vi "220221-VNA RP FLAT.vi"() -> ()   [LabVIEW 2021]
uses:
  b7fd31b3-4c8f-4ae8-a038-7c142e2eb182.vi
  <vilib>/Analysis/baseanly.llb/Mean (DBL).vi
  <vilib>/Utility/file.llb/Write Delimited Spreadsheet (DBL).vi
  <vilib>/Comparison/Equal/Equal Functor/Equal Functor.lvclass
  <vilib>/Analysis/NI_AALBase.lvlib
panel:
  in  "BTN VIEW PERSISTANCE":bool
  in  "Autoscale":bool
  in  "RP VNA SETTING":T1={"F start"=200000, "F stop"=2000500, "Sweep size"=1000, "Decimation"=5000, "F_corr"=0, "Ph_OUT1"=0, "Ph_OUT2"=0, "OUT_Lvl1"=32700, "OUT_Lvl2"=32700, "GPIO"=0}
  in  "Amplitude(1V)":dbl=0.3 format="%#_13g"
  out "RP CONNECT":bool
  in  "VOA Calibration cluster":cluster{"PUMP":dbl[], "PROBE":dbl[]}
  out "TRACK DATA REL NO SMOOTHING":dbl[][](array[numeric])
  out "TRACK DATA ABS NO SMOOTHING":dbl[][](array[numeric])
  in  "BTN SAVE TRACK":bool
  in  "BTN STOP TRACK":bool
  out "TRACK REPOSITERY":path
  out "TRACK DATA REL":dbl[][](array[numeric])
  out "TRACK DATA ABS":dbl[][](array[numeric])
  out "Track File List":path[](array[path])
  out "Track Repositery List":path[](array[path])
  out "CHANNEL CHOSEN":i32
  in  "TRACK-STOP":bool
  out "STATUS":string="STOP"
  out "track data":dbl[](array[numeric])=[495490.5081042979, 495481.56129759253, 495478.2328599854, 495479.84884744807, 495476.377462383, 495478.7819904735]
  out "Information tips":string
  in  "PANEL VNA":bool
  in  "PANEL TRACKING":bool
  in  "BTN STOP":bool
  in  "PANEL GENERAL SETTINGS":bool
  in  "PANEL TRACK SETTINGS":bool
  out "MAIN TAB":T2(tab)
  out "ACQ Indicator":bool
  in  "PUMP":dbl(slide)=100.0 min=0.0 max=100.0 step=0.1 scale=0.0..100.0
  in  "PROBE":dbl(slide)=100.0 min=0.0 max=100.0 step=0.1 scale=0.0..100.0
  in  "BTN RESET VNA":bool
  in  "SPAN":dbl=1900.0 format="%#5.1f"
  in  "STOP":dbl=2000.0 format="%#5.1f"
  in  "CENTER":dbl=1050.0 format="%#5.1f"
  in  "BTN AF VNA":bool
  out "MAGNITUDE/PHASE":cluster{cluster{dbl, dbl}[]}[](graph)
  in  "CHANNEL CHOICE VNA":T3(radio)
  in  "BTN Center to max":bool
  in  "BTN ZOOM-":bool
  in  "BTN ZOOM+":bool
  in  "START":dbl=200.0 format="%#5.1f"
  out "SPACING":dbl=1900.0 min=0.0 max=100.0 step=0.5 format="%#5.1f"
  in  "Points N°":i32=1000 min=600 max=5000 step=1 format="%#4.4g"
  in  "BTN LOOP VNA":bool
  in  "BTN RUN VNA":bool
  in  "BTN SAVE VNA":bool
  in  "Hide/Show track data channel":bool[](array[boolean])
  in  "BTN AUTOSAVE RAW DATA":bool=TRUE
  in  "COMMENTS":string
  in  "ASSAY NAME":string
  in  "DELAY AFTER SWITCH (s)":i32
  in  "N°POINTS TO DISPLAY":i32=200
  in  "DISPLAY OPTION":u16(ring) items=["Absolute frequency", "Relative frequency (ppm)"]
  in  "DELAY BETWEEN TRIG (s)":i32
  in  "AVERAGE/POINT":dbl=1.0
  out "LIVE TRACK":dbl[][](graph)
  out "CHANNELS IND TRACK":T3(radio)
  in  "BTN RUN TRACK":bool
  in  "TEMPORAL SMOOTHING":i32=15
  in  "BTN NEW TRACK":bool
  in  "BTN PAUSE TRACK":bool
  in  "CHANNELS PARAMETERS":T4(array[cluster])=[{"START 2"=200.0, "STOP 2"=2000.5, "CENTER 2"=1050.0, "SPAN 2"=1800.0, "CHANNEL TRACK ?"=FALSE, "PUMP"=100.0, "PROBE"=100.0, "Points N° 2"=1000, "SPACING 2"=100.0, "Parafit span"=0.0, "Parafit span type"=enum."Points N°"}, {"START 2"=200.0, "STOP 2"=2000.0, "CENTER 2"=1100.0, "SPAN 2"=1800.0, "CHANNEL TRACK ?"=FALSE, "PUMP"=100.0, "PROBE"=100.0, "Points N° 2"=1000, "SPACING 2"=1800.0, "Parafit span"=0.0, "Parafit span type"=enum."Points N°"}, {"START 2"=200.0, "STOP 2"=2000.0, "CENTER 2"=1100.0, "SPAN 2"=1800.0, "CHANNEL TRACK ?"=FALSE, "PUMP"=100.0, "PROBE"=100.0, "Points N° 2"=1000, "SPACING 2"=1800.0, "Parafit span"=0.0, "Parafit span type"=enum."Points N°"}, {"START 2"=200.0, "STOP 2"=2000.0, "CENTER 2"=1100.0, "SPAN 2"=1800.0, "CHANNEL TRACK ?"=FALSE, "PUMP"=100.0, "PROBE"=100.0, "Points N° 2"=1000, "SPACING 2"=1800.0, "Parafit span"=0.0, "Parafit span type"=enum."Points N°"}, {"START 2"=200.0, "STOP 2"=2000.0, "CENTER 2"=1100.0, "SPAN 2"=1800.0, "CHANNEL TRACK ?"=FALSE, "PUMP"=100.0, "PROBE"=100.0, "Points N° 2"=1000, "SPACING 2"=1800.0, "Parafit span"=0.0, "Parafit span type"=enum."Points N°"}, {"START 2"=200.0, "STOP 2"=2000.0, "CENTER 2"=1100.0, "SPAN 2"=1800.0, "CHANNEL TRACK ?"=FALSE, "PUMP"=100.0, "PROBE"=100.0, "Points N° 2"=1000, "SPACING 2"=1800.0, "Parafit span"=0.0, "Parafit span type"=enum."Points N°"}, {"START 2"=200.0, "STOP 2"=2000.0, "CENTER 2"=1100.0, "SPAN 2"=1800.0, "CHANNEL TRACK ?"=FALSE, "PUMP"=100.0, "PROBE"=100.0, "Points N° 2"=1000, "SPACING 2"=1800.0, "Parafit span"=0.0, "Parafit span type"=enum."Points N°"}, {"START 2"=200.0, "STOP 2"=2000.0, "CENTER 2"=1100.0, "SPAN 2"=1800.0, "CHANNEL TRACK ?"=FALSE, "PUMP"=100.0, "PROBE"=100.0, "Points N° 2"=1000, "SPACING 2"=1800.0, "Parafit span"=0.0, "Parafit span type"=enum."Points N°"}, {"START 2"=200.0, "STOP 2"=2000.0, "CENTER 2"=1100.0, "SPAN 2"=1800.0, "CHANNEL TRACK ?"=FALSE, "PUMP"=100.0, "PROBE"=100.0, "Points N° 2"=1000, "SPACING 2"=1800.0, "Parafit span"=0.0, "Parafit span type"=enum."Points N°"}, {"START 2"=200.0, "STOP 2"=2000.0, "CENTER 2"=1100.0, "SPAN 2"=1800.0, "CHANNEL TRACK ?"=FALSE, "PUMP"=100.0, "PROBE"=100.0, "Points N° 2"=1000, "SPACING 2"=1800.0, "Parafit span"=0.0, "Parafit span type"=enum."Points N°"}, {"START 2"=200.0, "STOP 2"=2000.0, "CENTER 2"=1100.0, "SPAN 2"=1800.0, "CHANNEL TRACK ?"=FALSE, "PUMP"=100.0, "PROBE"=100.0, "Points N° 2"=1000, "SPACING 2"=1800.0, "Parafit span"=0.0, "Parafit span type"=enum."Points N°"}, {"START 2"=200.0, "STOP 2"=2000.0, "CENTER 2"=1100.0, "SPAN 2"=1800.0, "CHANNEL TRACK ?"=FALSE, "PUMP"=100.0, "PROBE"=100.0, "Points N° 2"=1000, "SPACING 2"=1800.0, "Parafit span"=0.0, "Parafit span type"=enum."Points N°"}, {"START 2"=200.0, "STOP 2"=2000.0, "CENTER 2"=1100.0, "SPAN 2"=1800.0, "CHANNEL TRACK ?"=FALSE, "PUMP"=100.0, "PROBE"=100.0, "Points N° 2"=1000, "SPACING 2"=1800.0, "Parafit span"=0.0, "Parafit span type"=enum."Points N°"}, {"START 2"=200.0, "STOP 2"=2000.0, "CENTER 2"=1100.0, "SPAN 2"=1800.0, "CHANNEL TRACK ?"=FALSE, "PUMP"=100.0, "PROBE"=100.0, "Points N° 2"=1000, "SPACING 2"=1800.0, "Parafit span"=0.0, "Parafit span type"=enum."Points N°"}, {"START 2"=200.0, "STOP 2"=2000.0, "CENTER 2"=1100.0, "SPAN 2"=1800.0, "CHANNEL TRACK ?"=FALSE, "PUMP"=100.0, "PROBE"=100.0, "Points N° 2"=1000, "SPACING 2"=1800.0, "Parafit span"=0.0, "Parafit span type"=enum."Points N°"}, {"START 2"=200.0, "STOP 2"=2000.0, "CENTER 2"=1100.0, "SPAN 2"=1800.0, "CHANNEL TRACK ?"=FALSE, "PUMP"=100.0, "PROBE"=100.0, "Points N° 2"=1000, "SPACING 2"=1800.0, "Parafit span"=0.0, "Parafit span type"=enum."Points N°"}] {"SPACING 2" min=0.0 max=100.0 step=0.5; "Points N° 2" min=0 max=100 step=1; "PROBE" min=0.0 max=100.0 step=0.5; "PUMP" min=0.0 max=100.0 step=0.5}
  out "CHANNEL IND SETTINGS":T5(radio)
  in  "TRACK DATA PARAMETERS":cluster{"MAIN FOLDER":path}={"MAIN FOLDER"=path "C:/SensWay Data"}
  in  "SPECTRUM POST PROCESSING PARAMETERS":cluster{"N° SMOOTHING POINTS":i32}={"N° SMOOTHING POINTS"=50}
  in  "AUTOFOCUS PARAMETERS":cluster{"ITERATIONS":i32}={"ITERATIONS"=5}
  in  "CHANNELS":T6
  in  "NETWORK PARAMETERS":T7={"RP-IP 1"="192.168.0.3", "RP-IP 2"="192.168.0.4", "RP-MAC 1"="", "RP-MAC 2"=""}
  in  "PERSISTANCE DATA CLUSTER":T8
  in  "VNA DATA CLUSTER":T8
  in  "TRACK DATA CLUSTER":cluster{"CHANNEL":dbl, "KPI 1 TRACK":ext[]}
  out "LOOP ACT":bool
  out "RAW Freq table":dbl[](array[numeric])=[200000.0, 201802.3023023023, 203604.6046046046, 205406.9069069069, 207209.20920920922, 209011.51151151152, 210813.81381381382, 212616.1161161161, 214418.4184184184, 216220.7207207207, 218023.02302302304, 219825.32532532534, 221627.62762762763, 223429.92992992993, 225232.23223223223, 227034.53453453453, 228836.83683683682, 230639.13913913915, 232441.44144144145, 234243.74374374375, 236046.04604604605, 237848.34834834834, 239650.65065065064, 241452.95295295294, 243255.25525525527, 245057.55755755756, 246859.85985985986, 248662.16216216216, 250464.46446446446, 252266.76676676676, 254069.06906906905, 255871.37137137138, 257673.67367367368, 259475.97597597598, 261278.27827827827, 263080.5805805806, 264882.8828828829, 266685.18518518517, 268487.4874874875, 270289.7897897898, 272092.0920920921, 273894.39439439436, 275696.6966966967, 277498.998998999, 279301.3013013013, 281103.6036036036, 282905.9059059059, 284708.2082082082, 286510.51051051053, 288312.8128128128, 290115.1151151151, 291917.4174174174, 293719.7197197197, 295522.02202202205, 297324.3243243243, 299126.6266266266, 300928.9289289289, 302731.23123123124, 304533.5335335335, 306335.83583583584, 308138.1381381381, 309940.44044044043, 311742.74274274276, 313545.04504504503, 315347.34734734736, 317149.6496496496, 318951.95195195195, 320754.2542542543, 322556.55655655655, 324358.8588588588, 326161.16116116114, 327963.4634634635, 329765.76576576574, 331568.06806806807, 333370.37037037034, 335172.67267267266, 336974.974974975, 338777.27727727726, 340579.5795795796, 342381.88188188185, 344184.1841841842, 345986.4864864865, 347788.7887887888, 349591.09109109105, 351393.3933933934, 353195.6956956957, 354997.997997998, 356800.3003003003, 358602.60260260256, 360404.9049049049, 362207.2072072072, 364009.50950950955, 365811.8118118118, 367614.1141141141, 369416.4164164164, 371218.71871871874, 373021.021021021, 374823.3233233233, 376625.6256256256, 378427.9279279279, 380230.23023023026, 382032.5325325325, 383834.8348348348, 385637.1371371371, 387439.43943943945, 389241.7417417418, 391044.04404404404, 392846.3463463463, 394648.64864864864, 396450.95095095097, 398253.25325325324, 400055.5555555555, 401857.85785785783, 403660.16016016016, 405462.4624624625, 407264.76476476475, 409067.067067067, 410869.36936936935, 412671.6716716717, 414473.973973974, 416276.2762762763, 418078.57857857854, 419880.88088088087, 421683.1831831832, 423485.48548548546, 425287.7877877878, 427090.09009009006, 428892.3923923924, 430694.6946946947, 432496.996996997, 434299.29929929925, 436101.6016016016, 437903.9039039039, 439706.20620620623, 441508.5085085085, 443310.81081081077, 445113.1131131131, 446915.4154154154, 448717.7177177177, 450520.02002002, 452322.3223223223, 454124.6246246246, 455926.92692692694, 457729.2292292292, 459531.5315315315, 461333.8338338338, 463136.13613613613, 464938.4384384384, 466740.74074074073, 468543.04304304306, 470345.3453453453, 472147.64764764765, 473949.9499499499, 475752.25225225225, 477554.5545545545, 479356.85685685684, 481159.1591591592, 482961.46146146144, 484763.76376376377, 486566.06606606604, 488368.36836836836, 490170.67067067063, 491972.97297297296, 493775.2752752753, 495577.57757757755, 497379.8798798799, 499182.18218218215, 500984.4844844845, 502786.78678678675, 504589.0890890891, 506391.3913913914, 508193.69369369367, 509995.995995996, 511798.29829829826, 513600.6006006006, 515402.90290290286, 517205.2052052052, 519007.5075075075, 520809.8098098098, 522612.1121121121, 524414.4144144144, 526216.7167167168, 528019.0190190191, 529821.3213213213, 531623.6236236236, 533425.9259259258, 535228.2282282282, 537030.5305305305, 538832.8328328328, 540635.1351351351, 542437.4374374375, 544239.7397397398, 546042.042042042, 547844.3443443443, 549646.6466466465, 551448.9489489489, 553251.2512512512, 555053.5535535535, 556855.8558558559, 558658.1581581582, 560460.4604604605, 562262.7627627627, 564065.065065065, 565867.3673673674, 567669.6696696696, 569471.9719719719, 571274.2742742742, 573076.5765765766, 574878.8788788789, 576681.1811811812, 578483.4834834835, 580285.7857857858, 582088.0880880881, 583890.3903903903, 585692.6926926926, 587494.994994995, 589297.2972972973, 591099.5995995996, 592901.9019019019, 594704.2042042043, 596506.5065065065, 598308.8088088088, 600111.111111111, 601913.4134134133, 603715.7157157157, 605518.018018018, 607320.3203203203, 609122.6226226226, 610924.924924925, 612727.2272272272, 614529.5295295295, 616331.8318318318, 618134.134134134, 619936.4364364364, 621738.7387387387, 623541.041041041, 625343.3433433434, 627145.6456456457, 628947.947947948, 630750.2502502502, 632552.5525525525, 634354.8548548548, 636157.1571571571, 637959.4594594594, 639761.7617617617, 641564.0640640641, 643366.3663663664, 645168.6686686687, 646970.9709709709, 648773.2732732733, 650575.5755755756, 652377.8778778778, 654180.1801801801, 655982.4824824824, 657784.7847847848, 659587.0870870871, 661389.3893893894, 663191.6916916918, 664993.993993994, 666796.2962962963, 668598.5985985985, 670400.9009009008, 672203.2032032032, 674005.5055055055, 675807.8078078078, 677610.1101101101, 679412.4124124125, 681214.7147147147, 683017.017017017, 684819.3193193192, 686621.6216216215, 688423.9239239239, 690226.2262262262, 692028.5285285285, 693830.8308308308, 695633.1331331332, 697435.4354354354, 699237.7377377377, 701040.04004004, 702842.3423423423, 704644.6446446446, 706446.9469469469, 708249.2492492492, 710051.5515515516, 711853.8538538539, 713656.1561561562, 715458.4584584584, 717260.7607607607, 719063.063063063, 720865.3653653653, 722667.6676676676, 724469.9699699699, 726272.2722722723, 728074.5745745746, 729876.8768768768, 731679.1791791791, 733481.4814814815, 735283.7837837838, 737086.0860860861, 738888.3883883883, 740690.6906906907, 742492.992992993, 744295.2952952953, 746097.5975975975, 747899.8998998998, 749702.2022022022, 751504.5045045045, 753306.8068068068, 755109.109109109, 756911.4114114114, 758713.7137137137, 760516.016016016, 762318.3183183183, 764120.6206206206, 765922.9229229229, 767725.2252252252, 769527.5275275275, 771329.8298298299, 773132.1321321321, 774934.4344344344, 776736.7367367367, 778539.039039039, 780341.3413413413, 782143.6436436436, 783945.9459459459, 785748.2482482482, 787550.5505505506, 789352.8528528528, 791155.1551551551, 792957.4574574574, 794759.7597597598, 796562.0620620621, 798364.3643643643, 800166.6666666666, 801968.968968969, 803771.2712712713, 805573.5735735735, 807375.8758758758, 809178.1781781781, 810980.4804804805, 812782.7827827828, 814585.085085085, 816387.3873873873, 818189.6896896897, 819991.991991992, 821794.2942942943, 823596.5965965965, 825398.8988988989, 827201.2012012012, 829003.5035035035, 830805.8058058057, 832608.108108108, 834410.4104104104, 836212.7127127127, 838015.015015015, 839817.3173173172, 841619.6196196196, 843421.9219219219, 845224.2242242242, 847026.5265265265, 848828.8288288288, 850631.1311311311, 852433.4334334334, 854235.7357357357, 856038.0380380381, 857840.3403403403, 859642.6426426426, 861444.9449449449, 863247.2472472473, 865049.5495495495, 866851.8518518518, 868654.1541541541, 870456.4564564564, 872258.7587587588, 874061.061061061, 875863.3633633633, 877665.6656656656, 879467.967967968, 881270.2702702703, 883072.5725725725, 884874.8748748748, 886677.1771771772, 888479.4794794795, 890281.7817817817, 892084.084084084, 893886.3863863864, 895688.6886886887, 897490.990990991, 899293.2932932932, 901095.5955955955, 902897.8978978979, 904700.2002002002, 906502.5025025025, 908304.8048048047, 910107.1071071071, 911909.4094094094, 913711.7117117117, 915514.0140140139, 917316.3163163163, 919118.6186186186, 920920.9209209209, 922723.2232232232, 924525.5255255254, 926327.8278278278, 928130.1301301301, 929932.4324324324, 931734.7347347348, 933537.037037037, 935339.3393393393, 937141.6416416416, 938943.943943944, 940746.2462462463, 942548.5485485485, 944350.8508508508, 946153.1531531531, 947955.4554554555, 949757.7577577577, 951560.06006006, 953362.3623623623, 955164.6646646647, 956966.966966967, 958769.2692692692, 960571.5715715715, 962373.8738738738, 964176.1761761762, 965978.4784784785, 967780.7807807807, 969583.083083083, 971385.3853853854, 973187.6876876877, 974989.9899899899, 976792.2922922922, 978594.5945945946, 980396.8968968969, 982199.1991991992, 984001.5015015014, 985803.8038038037, 987606.1061061061, 989408.4084084084, 991210.7107107107, 993013.0130130129, 994815.3153153153, 996617.6176176176, 998419.9199199199, 1000222.2222222221, 1002024.5245245245, 1003826.8268268268, 1005629.1291291291, 1007431.4314314314, 1009233.7337337337, 1011036.036036036, 1012838.3383383383, 1014640.6406406406, 1016442.942942943, 1018245.2452452452, 1020047.5475475475, 1021849.8498498498, 1023652.1521521521, 1025454.4544544544, 1027256.7567567567, 1029059.059059059, 1030861.3613613613, 1032663.6636636637, 1034465.9659659659, 1036268.2682682682, 1038070.5705705705, 1039872.8728728729, 1041675.1751751752, 1043477.4774774774, 1045279.7797797797, 1047082.082082082, 1048884.3843843844, 1050686.6866866867, 1052488.988988989, 1054291.2912912914, 1056093.5935935937, 1057895.895895896, 1059698.198198198, 1061500.5005005004, 1063302.8028028028, 1065105.105105105, 1066907.4074074074, 1068709.7097097095, 1070512.0120120118, 1072314.3143143142, 1074116.6166166165, 1075918.9189189188, 1077721.2212212211, 1079523.5235235235, 1081325.8258258258, 1083128.1281281281, 1084930.4304304305, 1086732.7327327328, 1088535.035035035, 1090337.3373373374, 1092139.6396396398, 1093941.9419419419, 1095744.2442442442, 1097546.5465465465, 1099348.8488488488, 1101151.1511511512, 1102953.4534534533, 1104755.7557557556, 1106558.058058058, 1108360.3603603602, 1110162.6626626626, 1111964.964964965, 1113767.2672672672, 1115569.5695695695, 1117371.8718718719, 1119174.1741741742, 1120976.4764764765, 1122778.7787787789, 1124581.0810810812, 1126383.3833833835, 1128185.6856856856, 1129987.987987988, 1131790.2902902903, 1133592.5925925926, 1135394.894894895, 1137197.197197197, 1138999.4994994993, 1140801.8018018017, 1142604.104104104, 1144406.4064064063, 1146208.7087087086, 1148011.011011011, 1149813.3133133133, 1151615.6156156156, 1153417.917917918, 1155220.2202202203, 1157022.5225225226, 1158824.824824825, 1160627.1271271273, 1162429.4294294294, 1164231.7317317317, 1166034.034034034, 1167836.3363363363, 1169638.6386386384, 1171440.9409409408, 1173243.243243243, 1175045.5455455454, 1176847.8478478477, 1178650.15015015, 1180452.4524524524, 1182254.7547547547, 1184057.057057057, 1185859.3593593594, 1187661.6616616617, 1189463.963963964, 1191266.2662662663, 1193068.5685685687, 1194870.8708708708, 1196673.173173173, 1198475.4754754754, 1200277.7777777778, 1202080.08008008, 1203882.3823823822, 1205684.6846846845, 1207486.9869869868, 1209289.2892892892, 1211091.5915915915, 1212893.8938938938, 1214696.1961961961, 1216498.4984984985, 1218300.8008008008, 1220103.103103103, 1221905.4054054054, 1223707.7077077078, 1225510.01001001, 1227312.3123123124, 1229114.6146146145, 1230916.9169169168, 1232719.2192192192, 1234521.5215215215, 1236323.8238238238, 1238126.126126126, 1239928.4284284282, 1241730.7307307306, 1243533.033033033, 1245335.3353353352, 1247137.6376376376, 1248939.9399399399, 1250742.2422422422, 1252544.5445445445, 1254346.8468468469, 1256149.1491491492, 1257951.4514514515, 1259753.7537537536, 1261556.056056056, 1263358.3583583583, 1265160.6606606606, 1266962.962962963, 1268765.2652652652, 1270567.5675675676, 1272369.86986987, 1274172.1721721722, 1275974.4744744743, 1277776.7767767766, 1279579.079079079, 1281381.3813813813, 1283183.6836836836, 1284985.985985986, 1286788.2882882883, 1288590.5905905906, 1290392.892892893, 1292195.195195195, 1293997.4974974974, 1295799.7997997997, 1297602.102102102, 1299404.4044044043, 1301206.7067067067, 1303009.009009009, 1304811.3113113113, 1306613.6136136136, 1308415.915915916, 1310218.218218218, 1312020.5205205204, 1313822.8228228227, 1315625.125125125, 1317427.4274274274, 1319229.7297297297, 1321032.032032032, 1322834.3343343344, 1324636.6366366367, 1326438.9389389388, 1328241.241241241, 1330043.5435435434, 1331845.8458458458, 1333648.148148148, 1335450.4504504504, 1337252.7527527527, 1339055.055055055, 1340857.3573573574, 1342659.6596596597, 1344461.9619619618, 1346264.2642642641, 1348066.5665665665, 1349868.8688688688, 1351671.1711711711, 1353473.4734734735, 1355275.7757757758, 1357078.078078078, 1358880.3803803804, 1360682.6826826825, 1362484.9849849849, 1364287.2872872872, 1366089.5895895895, 1367891.8918918918, 1369694.1941941942, 1371496.4964964965, 1373298.7987987988, 1375101.1011011011, 1376903.4034034032, 1378705.7057057056, 1380508.008008008, 1382310.3103103102, 1384112.6126126125, 1385914.9149149149, 1387717.2172172172, 1389519.5195195195, 1391321.8218218219, 1393124.1241241242, 1394926.4264264263, 1396728.7287287286, 1398531.031031031, 1400333.3333333333, 1402135.6356356356, 1403937.937937938, 1405740.2402402402, 1407542.5425425426, 1409344.844844845, 1411147.147147147, 1412949.4494494493, 1414751.7517517516, 1416554.054054054, 1418356.3563563563, 1420158.6586586586, 1421960.960960961, 1423763.2632632633, 1425565.5655655656, 1427367.867867868, 1429170.17017017, 1430972.4724724723, 1432774.7747747747, 1434577.077077077, 1436379.3793793793, 1438181.6816816817, 1439983.983983984, 1441786.2862862863, 1443588.5885885886, 1445390.8908908907, 1447193.193193193, 1448995.4954954954, 1450797.7977977977, 1452600.1001001, 1454402.4024024024, 1456204.7047047047, 1458007.007007007, 1459809.3093093093, 1461611.6116116114, 1463413.9139139138, 1465216.216216216, 1467018.5185185184, 1468820.8208208208, 1470623.123123123, 1472425.4254254254, 1474227.7277277277, 1476030.03003003, 1477832.3323323324, 1479634.6346346345, 1481436.9369369368, 1483239.2392392391, 1485041.5415415415, 1486843.8438438438, 1488646.146146146, 1490448.4484484484, 1492250.7507507508, 1494053.053053053, 1495855.3553553552, 1497657.6576576575, 1499459.9599599598, 1501262.2622622622, 1503064.5645645645, 1504866.8668668668, 1506669.1691691692, 1508471.4714714715, 1510273.7737737738, 1512076.0760760761, 1513878.3783783782, 1515680.6806806806, 1517482.9829829829, 1519285.2852852852, 1521087.5875875875, 1522889.8898898899, 1524692.1921921922, 1526494.4944944945, 1528296.7967967968, 1530099.099099099, 1531901.4014014013, 1533703.7037037036, 1535506.006006006, 1537308.3083083082, 1539110.6106106106, 1540912.912912913, 1542715.2152152152, 1544517.5175175176, 1546319.8198198196, 1548122.122122122, 1549924.4244244243, 1551726.7267267266, 1553529.029029029, 1555331.3313313313, 1557133.6336336336, 1558935.935935936, 1560738.2382382383, 1562540.5405405406, 1564342.8428428427, 1566145.145145145, 1567947.4474474473, 1569749.7497497497, 1571552.052052052, 1573354.3543543543, 1575156.6566566566, 1576958.958958959, 1578761.2612612613, 1580563.5635635634, 1582365.8658658657, 1584168.168168168, 1585970.4704704704, 1587772.7727727727, 1589575.075075075, 1591377.3773773774, 1593179.6796796797, 1594981.981981982, 1596784.2842842843, 1598586.5865865864, 1600388.8888888888, 1602191.191191191, 1603993.4934934934, 1605795.7957957957, 1607598.098098098, 1609400.4004004004, 1611202.7027027027, 1613005.005005005, 1614807.3073073071, 1616609.6096096095, 1618411.9119119118, 1620214.2142142141, 1622016.5165165165, 1623818.8188188188, 1625621.121121121, 1627423.4234234234, 1629225.7257257258, 1631028.0280280279, 1632830.3303303302, 1634632.6326326325, 1636434.9349349348, 1638237.2372372372, 1640039.5395395395, 1641841.8418418418, 1643644.1441441441, 1645446.4464464465, 1647248.7487487488, 1649051.051051051, 1650853.3533533532, 1652655.6556556555, 1654457.9579579579, 1656260.2602602602, 1658062.5625625625, 1659864.8648648649, 1661667.1671671672, 1663469.4694694695, 1665271.7717717716, 1667074.074074074, 1668876.3763763763, 1670678.6786786786, 1672480.980980981, 1674283.2832832832, 1676085.5855855856, 1677887.887887888, 1679690.1901901902, 1681492.4924924925, 1683294.7947947946, 1685097.097097097, 1686899.3993993993, 1688701.7017017016, 1690504.004004004, 1692306.3063063063, 1694108.6086086086, 1695910.910910911, 1697713.2132132133, 1699515.5155155153, 1701317.8178178177, 1703120.12012012, 1704922.4224224223, 1706724.7247247247, 1708527.027027027, 1710329.3293293293, 1712131.6316316316, 1713933.933933934, 1715736.236236236, 1717538.5385385384, 1719340.8408408407, 1721143.143143143, 1722945.4454454454, 1724747.7477477477, 1726550.05005005, 1728352.3523523523, 1730154.6546546547, 1731956.956956957, 1733759.259259259, 1735561.5615615614, 1737363.8638638637, 1739166.166166166, 1740968.4684684684, 1742770.7707707707, 1744573.073073073, 1746375.3753753754, 1748177.6776776777, 1749979.9799799798, 1751782.2822822821, 1753584.5845845845, 1755386.8868868868, 1757189.189189189, 1758991.4914914914, 1760793.7937937938, 1762596.096096096, 1764398.3983983984, 1766200.7007007005, 1768003.0030030028, 1769805.3053053052, 1771607.6076076075, 1773409.9099099098, 1775212.2122122122, 1777014.5145145145, 1778816.8168168168, 1780619.1191191191, 1782421.4214214215, 1784223.7237237236, 1786026.0260260259, 1787828.3283283282, 1789630.6306306305, 1791432.9329329329, 1793235.2352352352, 1795037.5375375375, 1796839.8398398398, 1798642.1421421422, 1800444.4444444443, 1802246.7467467466, 1804049.049049049, 1805851.3513513512, 1807653.6536536536, 1809455.955955956, 1811258.2582582582, 1813060.5605605606, 1814862.8628628629, 1816665.1651651652, 1818467.4674674673, 1820269.7697697696, 1822072.072072072, 1823874.3743743743, 1825676.6766766766, 1827478.978978979, 1829281.2812812813, 1831083.5835835836, 1832885.885885886, 1834688.188188188, 1836490.4904904903, 1838292.7927927927, 1840095.095095095, 1841897.3973973973, 1843699.6996996996, 1845502.002002002, 1847304.3043043043, 1849106.6066066066, 1850908.9089089087, 1852711.211211211, 1854513.5135135134, 1856315.8158158157, 1858118.118118118, 1859920.4204204204, 1861722.7227227227, 1863525.025025025, 1865327.3273273273, 1867129.6296296297, 1868931.9319319318, 1870734.234234234, 1872536.5365365364, 1874338.8388388387, 1876141.141141141, 1877943.4434434434, 1879745.7457457457, 1881548.048048048, 1883350.3503503504, 1885152.6526526525, 1886954.9549549548, 1888757.2572572571, 1890559.5595595594, 1892361.8618618618, 1894164.164164164, 1895966.4664664664, 1897768.7687687688, 1899571.071071071, 1901373.3733733734, 1903175.6756756755, 1904977.9779779778, 1906780.2802802802, 1908582.5825825825, 1910384.8848848848, 1912187.1871871871, 1913989.4894894895, 1915791.7917917918, 1917594.0940940941, 1919396.3963963962, 1921198.6986986985, 1923001.0010010009, 1924803.3033033032, 1926605.6056056055, 1928407.9079079079, 1930210.2102102102, 1932012.5125125125, 1933814.8148148148, 1935617.117117117, 1937419.4194194193, 1939221.7217217216, 1941024.024024024, 1942826.3263263262, 1944628.6286286286, 1946430.930930931, 1948233.2332332332, 1950035.5355355355, 1951837.8378378379, 1953640.14014014, 1955442.4424424423, 1957244.7447447446, 1959047.047047047, 1960849.3493493493, 1962651.6516516516, 1964453.953953954, 1966256.2562562563, 1968058.5585585586, 1969860.8608608607, 1971663.163163163, 1973465.4654654653, 1975267.7677677677, 1977070.07007007, 1978872.3723723723, 1980674.6746746746, 1982476.976976977, 1984279.2792792793, 1986081.5815815816, 1987883.8838838837, 1989686.186186186, 1991488.4884884884, 1993290.7907907907, 1995093.093093093, 1996895.3953953953, 1998697.6976976977, 2000500.0]
  in  "ENABLE INTERNAL MODULATION":bool=TRUE
  in  "VNA DATA CLUSTER TBL":T9(array[cluster])=[{"CHANNEL"=0.0, "FREQUENCY TABLE"=[0.0], "MAGNITUDE TABLE"=[0.0], "PHASE TABLE"=[0.0]}, {"CHANNEL"=1.0, "FREQUENCY TABLE"=[], "MAGNITUDE TABLE"=[], "PHASE TABLE"=[]}, {"CHANNEL"=2.0, "FREQUENCY TABLE"=[], "MAGNITUDE TABLE"=[], "PHASE TABLE"=[]}, {"CHANNEL"=3.0, "FREQUENCY TABLE"=[], "MAGNITUDE TABLE"=[], "PHASE TABLE"=[]}, {"CHANNEL"=4.0, "FREQUENCY TABLE"=[], "MAGNITUDE TABLE"=[], "PHASE TABLE"=[]}, {"CHANNEL"=5.0, "FREQUENCY TABLE"=[], "MAGNITUDE TABLE"=[], "PHASE TABLE"=[]}, {"CHANNEL"=6.0, "FREQUENCY TABLE"=[], "MAGNITUDE TABLE"=[], "PHASE TABLE"=[]}, {"CHANNEL"=7.0, "FREQUENCY TABLE"=[], "MAGNITUDE TABLE"=[], "PHASE TABLE"=[]}, {"CHANNEL"=8.0, "FREQUENCY TABLE"=[], "MAGNITUDE TABLE"=[], "PHASE TABLE"=[]}, {"CHANNEL"=9.0, "FREQUENCY TABLE"=[], "MAGNITUDE TABLE"=[], "PHASE TABLE"=[]}, {"CHANNEL"=10.0, "FREQUENCY TABLE"=[], "MAGNITUDE TABLE"=[], "PHASE TABLE"=[]}, {"CHANNEL"=11.0, "FREQUENCY TABLE"=[], "MAGNITUDE TABLE"=[], "PHASE TABLE"=[]}, {"CHANNEL"=12.0, "FREQUENCY TABLE"=[], "MAGNITUDE TABLE"=[], "PHASE TABLE"=[]}, {"CHANNEL"=13.0, "FREQUENCY TABLE"=[], "MAGNITUDE TABLE"=[], "PHASE TABLE"=[]}, {"CHANNEL"=14.0, "FREQUENCY TABLE"=[], "MAGNITUDE TABLE"=[], "PHASE TABLE"=[]}, {"CHANNEL"=15.0, "FREQUENCY TABLE"=[], "MAGNITUDE TABLE"=[], "PHASE TABLE"=[]}]
  in  "TRACK DATA CLUSTER TBL":cluster{"CHANNEL":dbl, "KPI 1 TRACK":ext[]}[](array[cluster])
  in  "VNA Settings cluster":T10={"START 2"=200.0, "STOP 2"=2000.5, "CENTER 2"=1050.0, "SPAN 2"=1901.0, "CHANNEL TRACK ?"=FALSE, "PUMP"=100.0, "PROBE"=100.0, "Points N° 2"=1000, "SPACING 2"=1901.0, "Parafit span"=0.0, "Parafit span type"=enum."Points N°"} {"SPACING 2" min=0.0 max=100.0 step=0.5; "Points N° 2" min=0 max=100 step=1; "PROBE" min=0.0 max=100.0 step=0.5; "PUMP" min=0.0 max=100.0 step=0.5}
  # "E"
  # "POINTS"
  # "SPACING"
  # "TRACK ?"
  # "START"
  # "STOP"
  # "CENTER"
  # "SPAN"
  # "PROBE"
  # "PUMP"
  # "PARABOLIC FIT SPAN"
  # "DATA ENTRY"
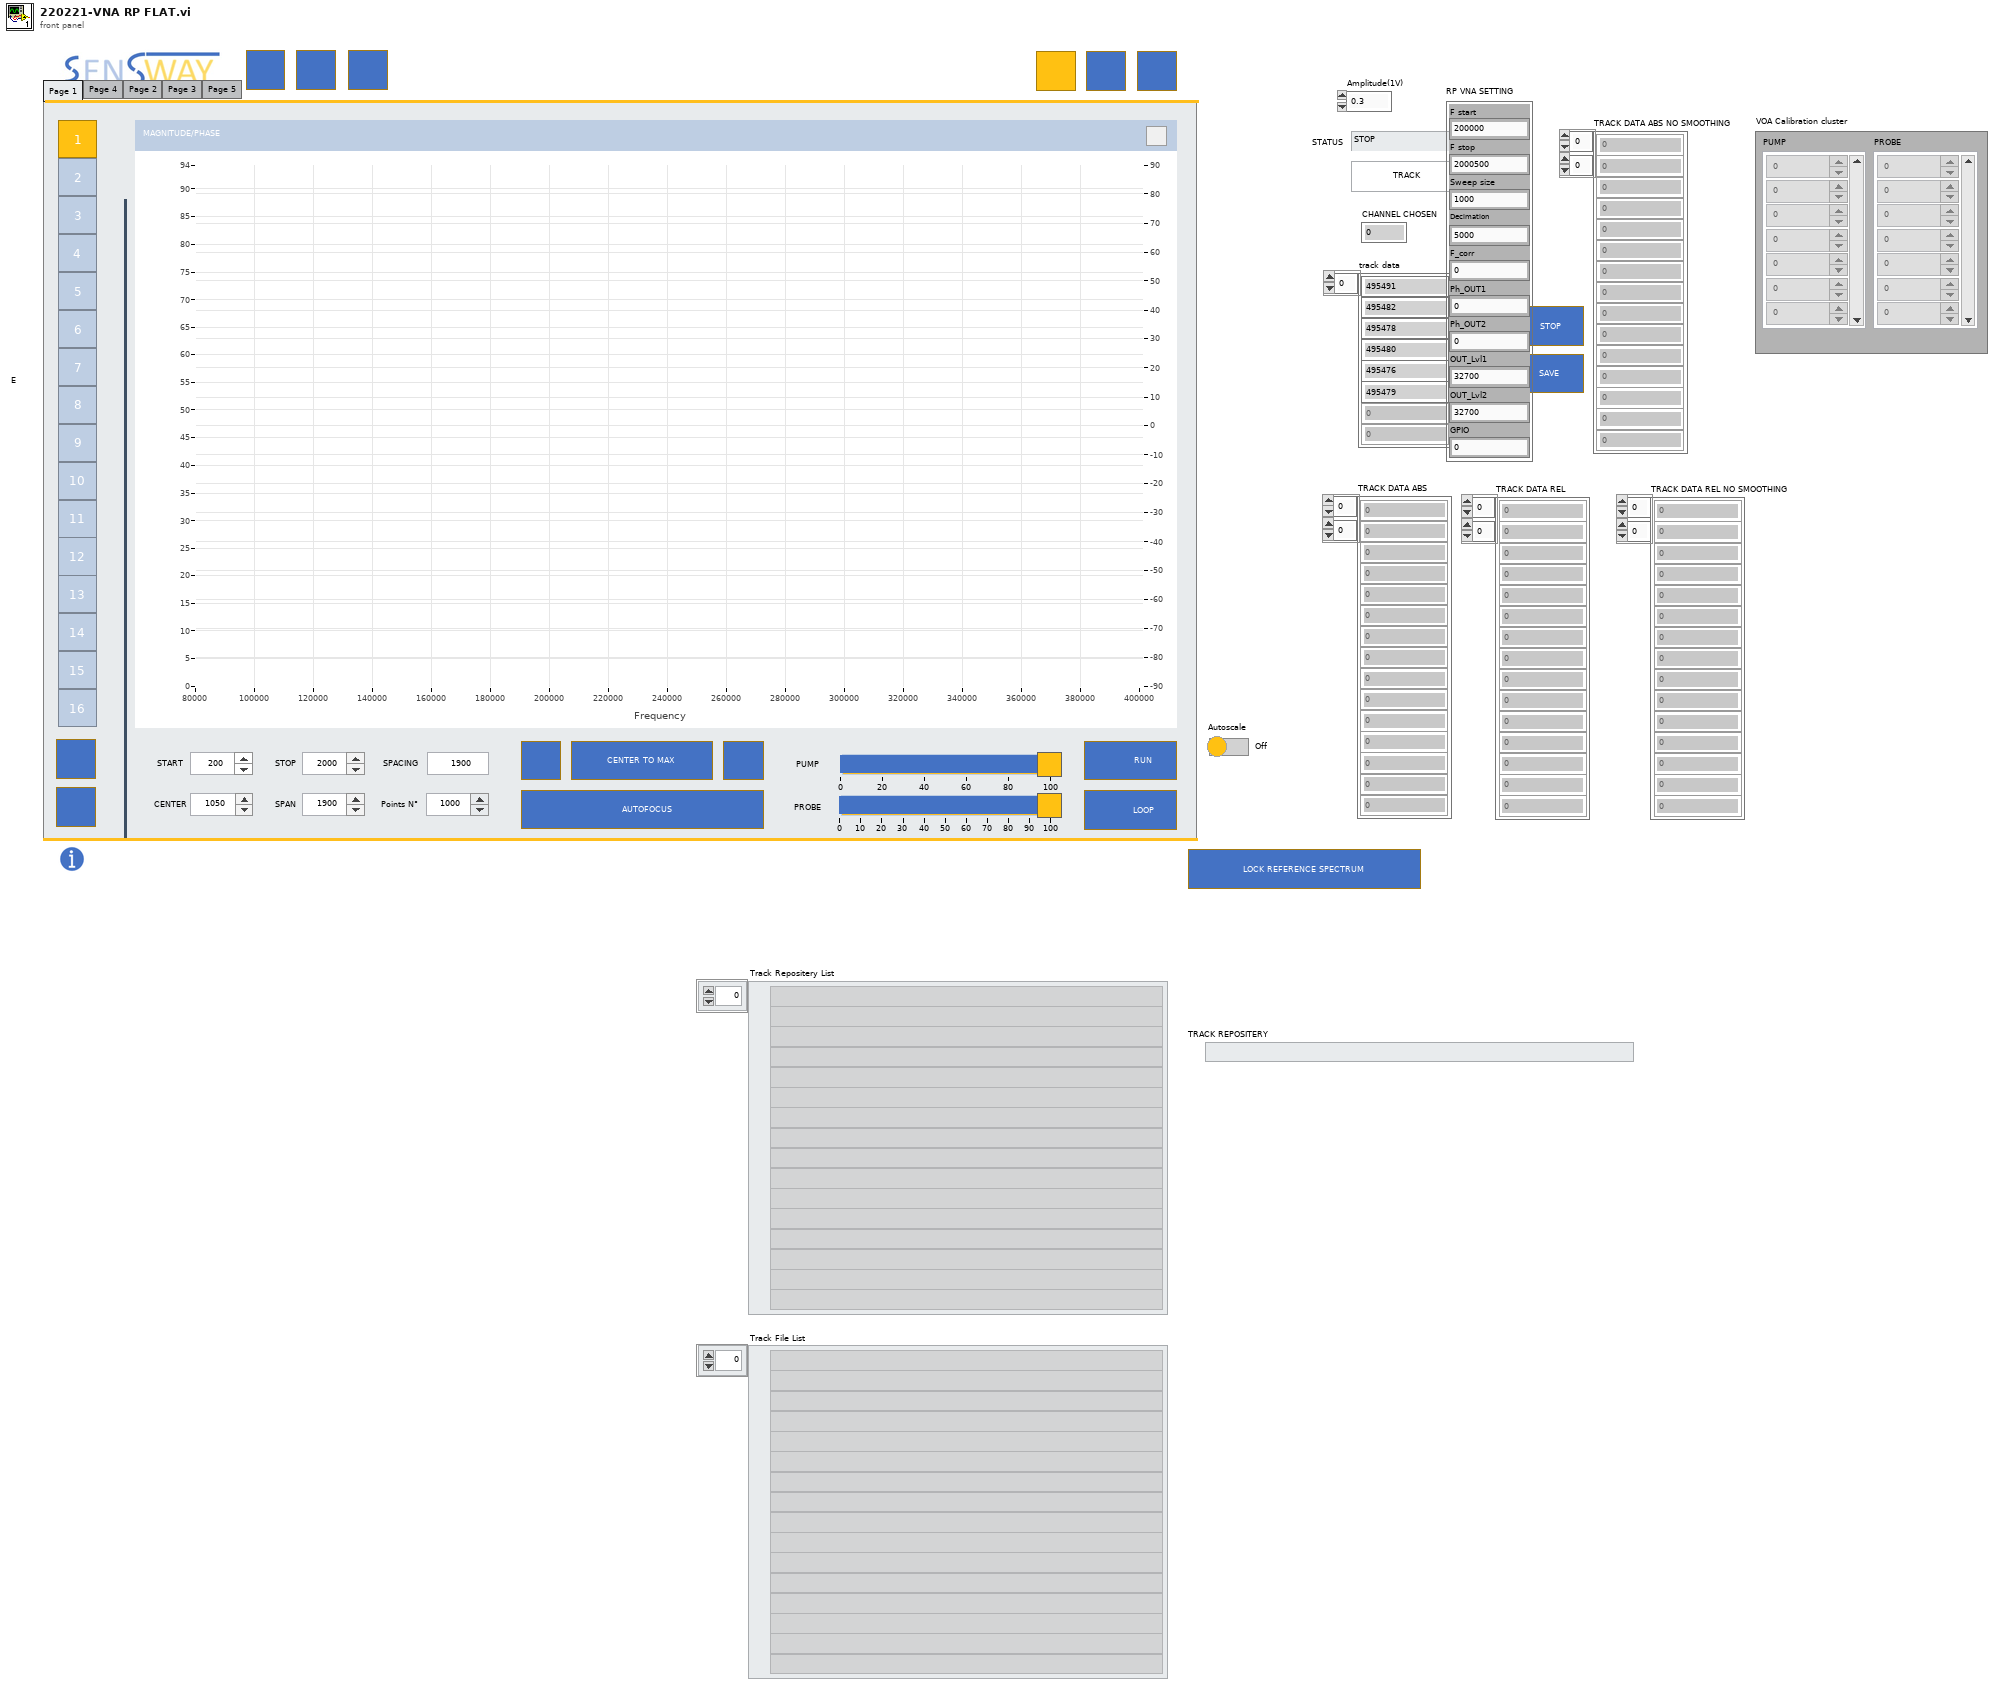
[diagram p1: front panel]
types:
  T1 = cluster{"F start":u32, "F stop":u32, "Sweep size":u32, "Decimation":u32, "F_corr":u32, "Ph_OUT1":u32, "Ph_OUT2":u32, "OUT_Lvl1":u32, "OUT_Lvl2":u32, "GPIO":u32}
  T2 = enum32{"Page 1", "Page 4", "Page 2", "Page 3", "Page 5"}
  T3 = enum32{"Button 1", "Button 2", "Button 3", "Sélection radio 4", "Sélection radio 5", "Sélection radio 6", "Sélection radio 7", "Sélection radio 8", "Sélection radio 9", "Sélection radio 10", "Sélection radio 11", "Sélection radio 12", "Sélection radio 13", "Sélection radio 14", "Sélection radio 15", "Sélection radio 16"}
  T4 = cluster{"START 2":dbl, "STOP 2":dbl, "CENTER 2":dbl, "SPAN 2":dbl, "CHANNEL TRACK ?":bool, "PUMP":dbl, "PROBE":dbl, "Points N° 2":i32, "SPACING 2":dbl, "Parafit span":dbl, "Parafit span type":enum16{"Points N°", "Frequency", "Span %"}}[]
  T5 = enum32{"No Selection", "Button 1", "Button 2", "Button 3", "Sélection radio 4", "Sélection radio 5", "Sélection radio 6", "Sélection radio 7", "Sélection radio 8", "Sélection radio 9", "Sélection radio 10", "Sélection radio 11", "Sélection radio 12", "Sélection radio 13", "Sélection radio 14", "Sélection radio 15", "Sélection radio 16"}
  T6 = cluster{"CHANNEL 1":bool, "CHANNEL 2":bool, "CHANNEL 3":bool, "CHANNEL 4":bool, "CHANNEL 5":bool, "CHANNEL 6":bool, "CHANNEL 7":bool, "CHANNEL 8":bool, "CHANNEL 9":bool, "CHANNEL 10":bool, "CHANNEL 11":bool, "CHANNEL 12":bool, "CHANNEL 13":bool, "CHANNEL 14":bool, "CHANNEL 15":bool, "CHANNEL 16":bool}
  T7 = cluster{"RP-IP 1":string, "RP-IP 2":string, "RP-MAC 1":string, "RP-MAC 2":string}
  T8 = cluster{"CHANNEL":dbl, "FREQUENCY TABLE":ext[], "MAGNITUDE TABLE":ext[], "PHASE TABLE":ext[]}
  T9 = cluster{"CHANNEL":dbl, "FREQUENCY TABLE":ext[], "MAGNITUDE TABLE":ext[], "PHASE TABLE":ext[]}[]
  T10 = cluster{"START 2":dbl, "STOP 2":dbl, "CENTER 2":dbl, "SPAN 2":dbl, "CHANNEL TRACK ?":bool, "PUMP":dbl, "PROBE":dbl, "Points N° 2":i32, "SPACING 2":dbl, "Parafit span":dbl, "Parafit span type":enum16{"Points N°", "Frequency", "Span %"}}
  T11 = enum16{"Freq start", "Freq stop", "Sweep size", "Decimation rate", "Freq corr", "Phase output 1", "Phase output 2", "Output level 1", "Output level 2", "GPIO", "SWEEP START"}
  T12 = cluster{"Numeric Control":ext, "Numeric Control":ext}[]
  T13 = cluster{cluster{"Numeric Control":ext, "Numeric Control":ext}[]}
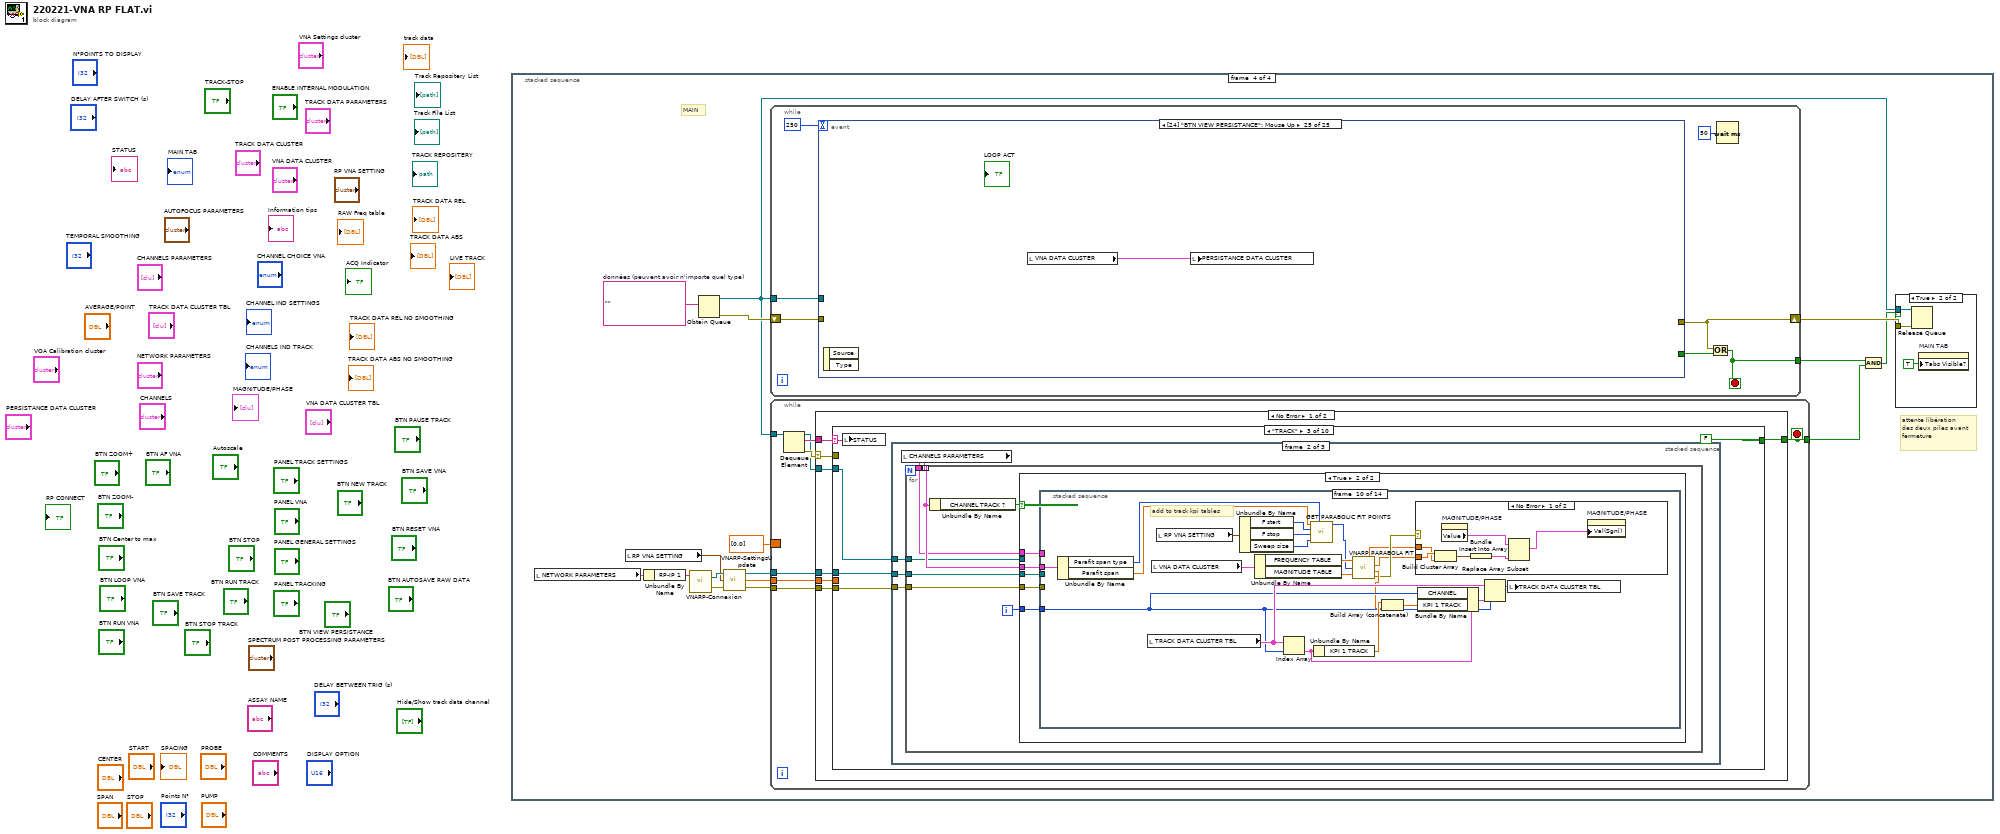
[diagram p0: block diagram]
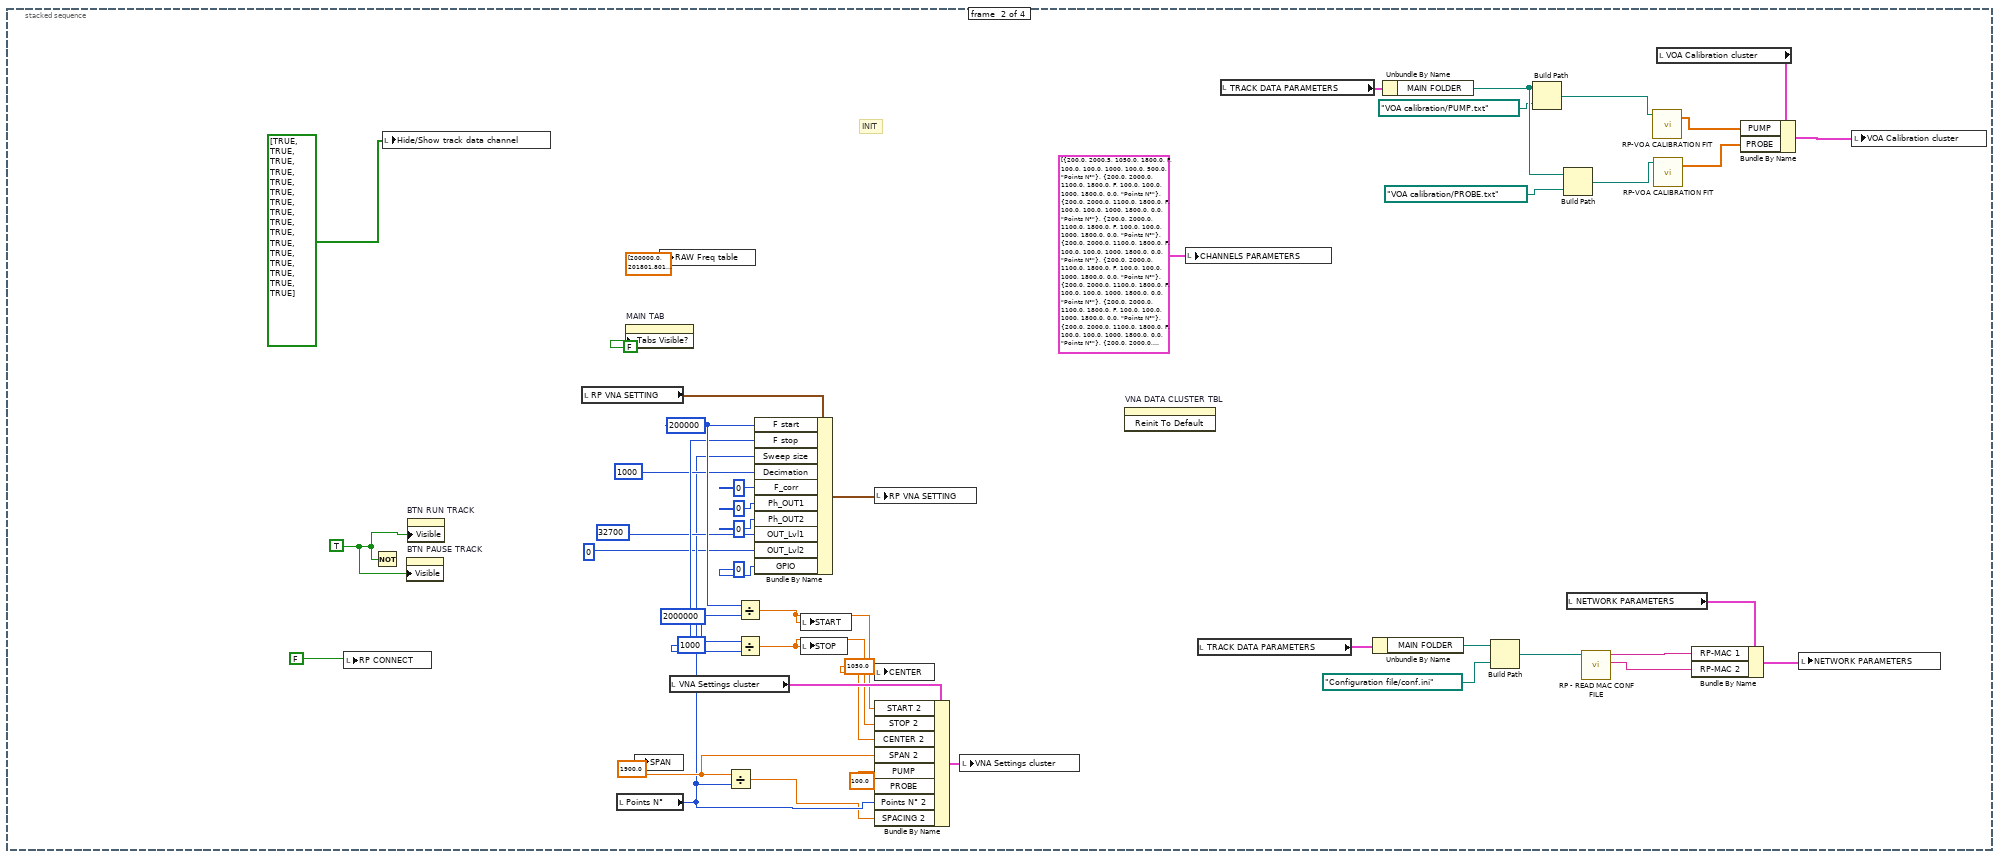
[diagram p3: hidden frame]
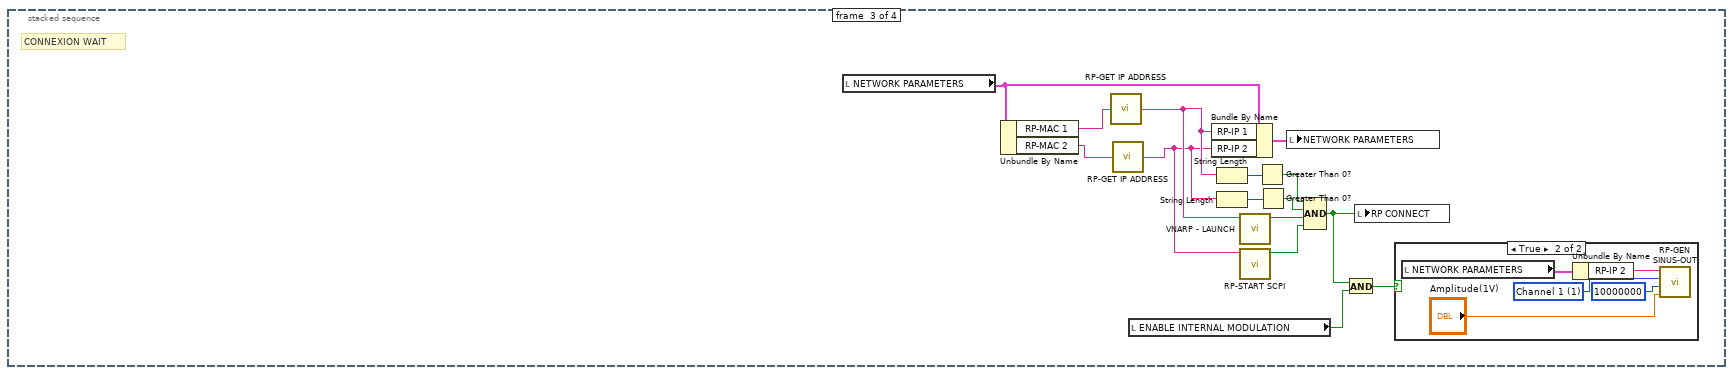
[diagram p4: hidden frame]
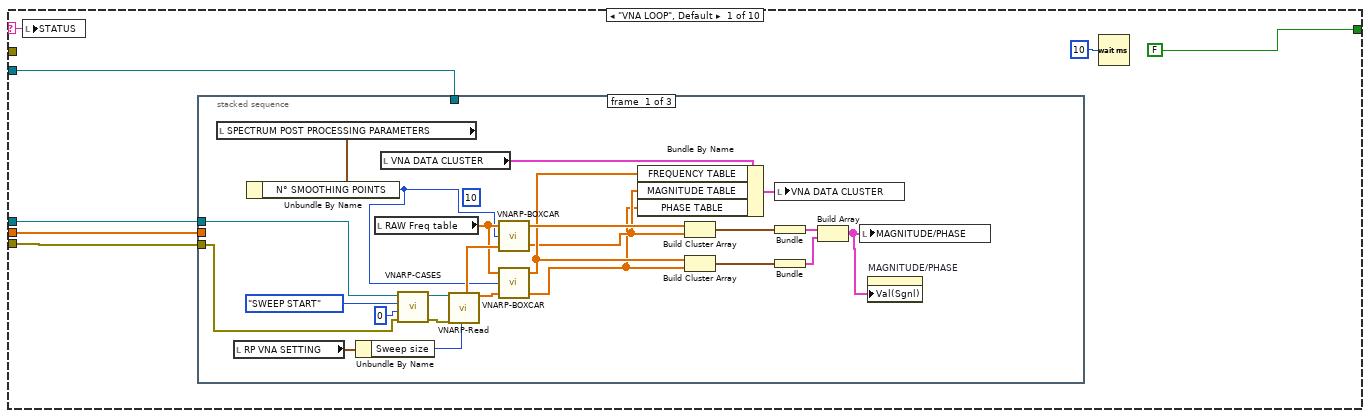
[diagram p7: hidden frame]
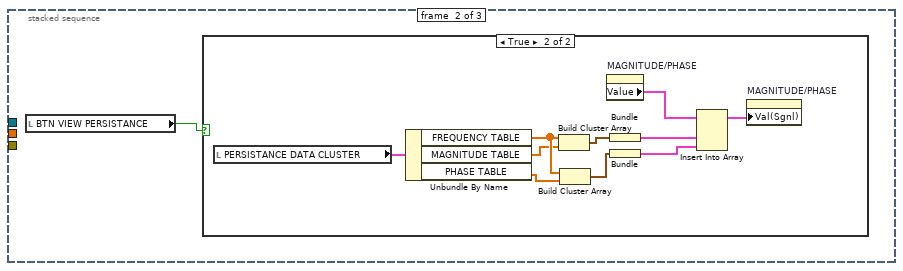
[diagram p8: hidden frame]
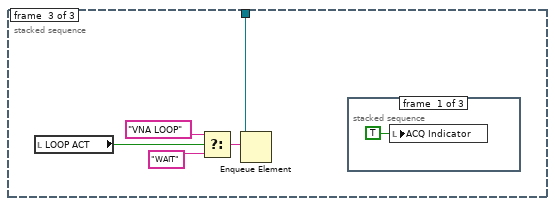
[diagram p10: hidden frame]
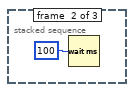
[diagram p11: hidden frame]
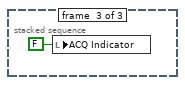
[diagram p12: hidden frame]
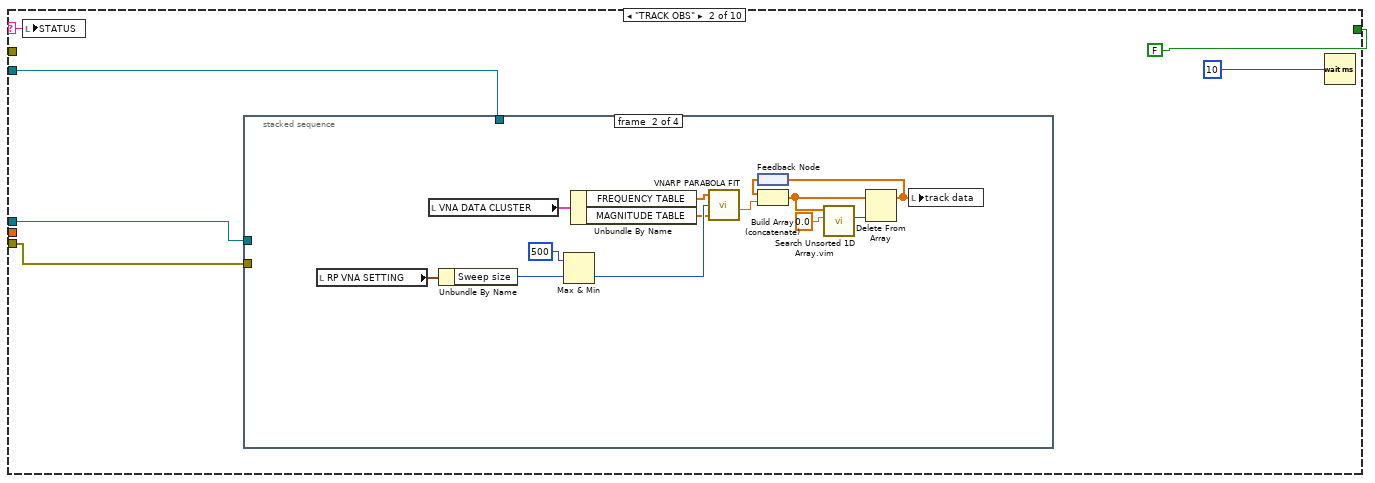
[diagram p13: hidden frame]
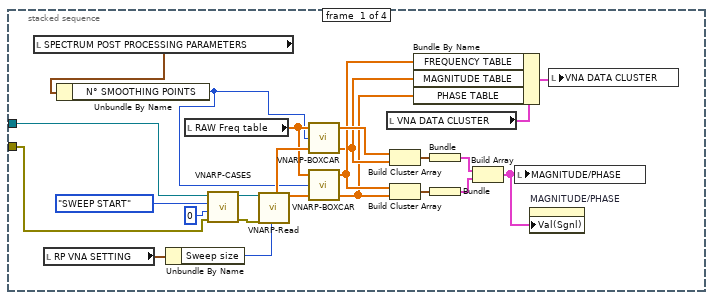
[diagram p14: hidden frame]
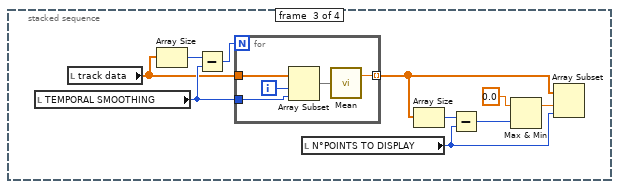
[diagram p15: hidden frame]
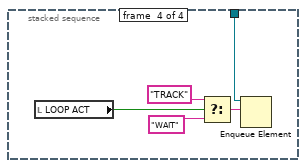
[diagram p16: hidden frame]
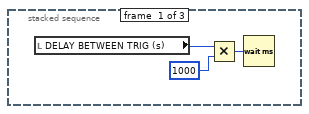
[diagram p17: hidden frame]
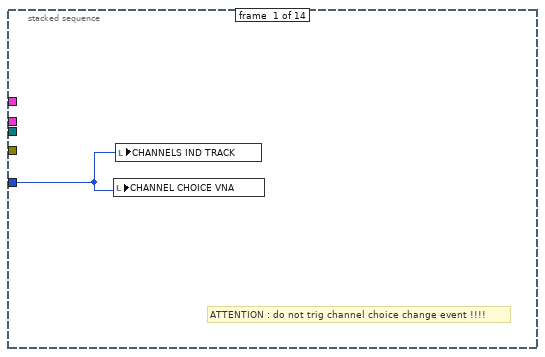
[diagram p19: hidden frame]
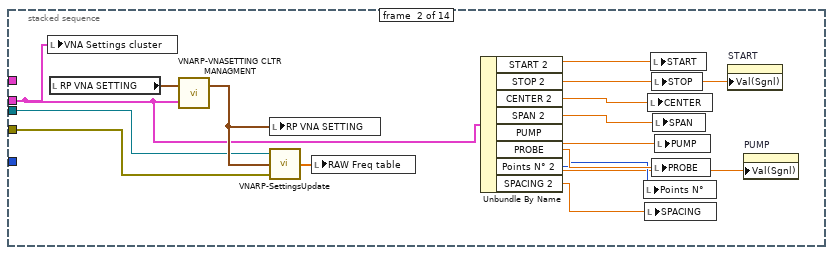
[diagram p20: hidden frame]
diagram:
  n1 = stacked-sequence {
    frame #0 {
    }
    frame #1 {
      w23 = TRUE ("x")
      w24 = 100.0 ("PUMP")
      w27 = 1900.0 ("Center")
      w28 = 1050.0 ("Center")
      w43 = u32 1000 ("Decimation")
      w41 = u32 2000000 ("Decimation")
      w42 = u32 200000 ("Decimation")
      # "INIT"
      n2 = local write "RP CONNECT"(FALSE) -> ()
      n3 = Not(x=w23) -> ()  [unwired: 1 out]
      n4 = local write "Hide/Show track data channel"(bool[] [TRUE, TRUE, TRUE, TRUE, TRUE, TRUE, TRUE, TRUE, TRUE, TRUE, TRUE, TRUE, TRUE, TRUE, TRUE, TRUE] ("Hide/Show track data channel")) -> ()
      n5 = property on="BTN PAUSE TRACK" class="Bool (strict)"("Visible"=w23) -> ()  [unwired: 2 in, 2 out]
      n6 = property on="BTN RUN TRACK" class="Bool (strict)"("Visible"=w23) -> ()  [unwired: 2 in, 2 out]
      n7 = local read "RP VNA SETTING"() -> (w45:T1)
      n8 = local read "Points N°"() -> (w26:i32)
      n9 = property on="MAIN TAB" class="TabCtl (strict)"("Tabs Visible?"=FALSE ("Onglets visibles ?")) -> ()  [unwired: 2 in, 2 out]
      n10 = local write "SPAN"(w27) -> ()
      n11 = local write "RAW Freq table"(dbl[] [200000.0, 201801.8018018018, 203603.6036036036, 205405.4054054054, 207207.20720720722, 209009.009009009, 210810.8108108108, 212612.6126126126, 214414.4144144144, 216216.2162162162, 218018.01801801802, 219819.81981981982, 221621.62162162163, 223423.42342342343, 225225.22522522524, 227027.02702702704, 228828.82882882882, 230630.63063063062, 232432.43243243243, 234234.23423423423, 236036.03603603604, 237837.83783783784, 239639.63963963964, 241441.44144144145, 243243.24324324325, 245045.04504504503, 246846.84684684683, 248648.64864864864, 250450.45045045044, 252252.25225225225, 254054.05405405405, 255855.85585585586, 257657.65765765766, 259459.45945945947, 261261.26126126124, 263063.0630630631, 264864.86486486485, 266666.6666666666, 268468.46846846846, 270270.2702702703, 272072.0720720721, 273873.87387387385, 275675.6756756757, 277477.47747747746, 279279.2792792793, 281081.08108108107, 282882.8828828829, 284684.6846846847, 286486.4864864865, 288288.2882882883, 290090.09009009006, 291891.8918918919, 293693.69369369367, 295495.4954954955, 297297.2972972973, 299099.0990990991, 300900.9009009009, 302702.7027027027, 304504.5045045045, 306306.3063063063, 308108.1081081081, 309909.90990990994, 311711.7117117117, 313513.5135135135, 315315.3153153153, 317117.1171171171, 318918.91891891893, 320720.7207207207, 322522.5225225225, 324324.3243243243, 326126.12612612615, 327927.9279279279, 329729.7297297297, 331531.53153153154, 333333.3333333333, 335135.13513513515, 336936.9369369369, 338738.7387387387, 340540.54054054053, 342342.34234234237, 344144.14414414414, 345945.9459459459, 347747.74774774775, 349549.5495495496, 351351.35135135136, 353153.15315315314, 354954.9549549549, 356756.75675675675, 358558.5585585586, 360360.36036036036, 362162.16216216213, 363963.96396396396, 365765.7657657658, 367567.5675675676, 369369.36936936935, 371171.1711711711, 372972.97297297296, 374774.7747747748, 376576.57657657657, 378378.37837837834, 380180.1801801802, 381981.981981982, 383783.7837837838, 385585.58558558556, 387387.38738738734, 389189.1891891892, 390990.990990991, 392792.7927927928, 394594.59459459456, 396396.3963963964, 398198.1981981982, 400000.0, 401801.8018018018, 403603.6036036036, 405405.4054054054, 407207.2072072072, 409009.009009009, 410810.81081081077, 412612.6126126126, 414414.41441441444, 416216.2162162162, 418018.018018018, 419819.8198198198, 421621.62162162166, 423423.42342342343, 425225.2252252252, 427027.027027027, 428828.8288288288, 430630.63063063065, 432432.4324324324, 434234.2342342342, 436036.03603603604, 437837.83783783787, 439639.63963963964, 441441.4414414414, 443243.2432432432, 445045.04504504503, 446846.84684684686, 448648.64864864864, 450450.4504504504, 452252.25225225225, 454054.0540540541, 455855.85585585586, 457657.65765765763, 459459.4594594594, 461261.26126126124, 463063.0630630631, 464864.86486486485, 466666.6666666666, 468468.46846846846, 470270.27027027024, 472072.0720720721, 473873.87387387385, 475675.6756756757, 477477.47747747746, 479279.2792792793, 481081.08108108107, 482882.8828828829, 484684.6846846847, 486486.48648648645, 488288.2882882883, 490090.09009009006, 491891.8918918919, 493693.69369369367, 495495.4954954955, 497297.2972972973, 499099.0990990991, 500900.9009009009, 502702.70270270266, 504504.5045045045, 506306.3063063063, 508108.1081081081, 509909.9099099099, 511711.7117117117, 513513.5135135135, 515315.3153153153, 517117.1171171171, 518918.91891891893, 520720.7207207207, 522522.5225225225, 524324.3243243243, 526126.1261261262, 527927.9279279279, 529729.7297297297, 531531.5315315316, 533333.3333333333, 535135.1351351351, 536936.9369369369, 538738.7387387387, 540540.5405405406, 542342.3423423423, 544144.1441441441, 545945.9459459459, 547747.7477477477, 549549.5495495496, 551351.3513513514, 553153.1531531531, 554954.9549549549, 556756.7567567567, 558558.5585585586, 560360.3603603604, 562162.1621621621, 563963.963963964, 565765.7657657657, 567567.5675675676, 569369.3693693693, 571171.1711711711, 572972.972972973, 574774.7747747747, 576576.5765765766, 578378.3783783783, 580180.1801801801, 581981.981981982, 583783.7837837838, 585585.5855855856, 587387.3873873875, 589189.1891891891, 590990.990990991, 592792.7927927928, 594594.5945945946, 596396.3963963964, 598198.1981981981, 600000.0, 601801.8018018018, 603603.6036036036, 605405.4054054054, 607207.2072072072, 609009.009009009, 610810.8108108108, 612612.6126126125, 614414.4144144144, 616216.2162162162, 618018.018018018, 619819.8198198199, 621621.6216216215, 623423.4234234234, 625225.2252252252, 627027.027027027, 628828.8288288289, 630630.6306306305, 632432.4324324324, 634234.2342342342, 636036.036036036, 637837.8378378379, 639639.6396396396, 641441.4414414414, 643243.2432432433, 645045.045045045, 646846.8468468469, 648648.6486486486, 650450.4504504504, 652252.2522522523, 654054.054054054, 655855.8558558559, 657657.6576576576, 659459.4594594594, 661261.2612612613, 663063.063063063, 664864.8648648649, 666666.6666666666, 668468.4684684684, 670270.2702702703, 672072.0720720721, 673873.8738738738, 675675.6756756757, 677477.4774774774, 679279.2792792793, 681081.0810810811, 682882.8828828828, 684684.6846846847, 686486.4864864864, 688288.2882882883, 690090.0900900901, 691891.8918918918, 693693.6936936937, 695495.4954954955, 697297.2972972973, 699099.099099099, 700900.9009009008, 702702.7027027027, 704504.5045045045, 706306.3063063063, 708108.1081081082, 709909.9099099098, 711711.7117117117, 713513.5135135135, 715315.3153153153, 717117.1171171172, 718918.9189189188, 720720.7207207207, 722522.5225225225, 724324.3243243243, 726126.1261261262, 727927.9279279279, 729729.7297297297, 731531.5315315315, 733333.3333333333, 735135.1351351351, 736936.9369369369, 738738.7387387387, 740540.5405405405, 742342.3423423424, 744144.1441441441, 745945.9459459459, 747747.7477477477, 749549.5495495496, 751351.3513513514, 753153.1531531531, 754954.9549549549, 756756.7567567567, 758558.5585585586, 760360.3603603604, 762162.1621621621, 763963.9639639639, 765765.7657657658, 767567.5675675676, 769369.3693693693, 771171.1711711711, 772972.9729729729, 774774.7747747748, 776576.5765765766, 778378.3783783783, 780180.1801801801, 781981.981981982, 783783.7837837838, 785585.5855855856, 787387.3873873873, 789189.1891891891, 790990.990990991, 792792.7927927928, 794594.5945945946, 796396.3963963963, 798198.1981981982, 800000.0, 801801.8018018018, 803603.6036036036, 805405.4054054053, 807207.2072072072, 809009.009009009, 810810.8108108108, 812612.6126126125, 814414.4144144144, 816216.2162162162, 818018.018018018, 819819.8198198198, 821621.6216216215, 823423.4234234234, 825225.2252252252, 827027.027027027, 828828.8288288288, 830630.6306306307, 832432.4324324324, 834234.2342342342, 836036.036036036, 837837.8378378379, 839639.6396396396, 841441.4414414414, 843243.2432432432, 845045.045045045, 846846.8468468469, 848648.6486486486, 850450.4504504504, 852252.2522522522, 854054.0540540541, 855855.8558558559, 857657.6576576576, 859459.4594594594, 861261.2612612612, 863063.0630630631, 864864.8648648649, 866666.6666666666, 868468.4684684684, 870270.2702702703, 872072.0720720721, 873873.8738738738, 875675.6756756756, 877477.4774774774, 879279.2792792793, 881081.0810810811, 882882.8828828828, 884684.6846846846, 886486.4864864865, 888288.2882882883, 890090.0900900901, 891891.8918918918, 893693.6936936936, 895495.4954954955, 897297.2972972973, 899099.099099099, 900900.9009009008, 902702.7027027027, 904504.5045045045, 906306.3063063063, 908108.108108108, 909909.9099099098, 911711.7117117117, 913513.5135135135, 915315.3153153153, 917117.117117117, 918918.9189189189, 920720.7207207207, 922522.5225225225, 924324.3243243243, 926126.1261261262, 927927.9279279279, 929729.7297297297, 931531.5315315315, 933333.3333333333, 935135.1351351351, 936936.9369369369, 938738.7387387387, 940540.5405405405, 942342.3423423424, 944144.1441441441, 945945.9459459459, 947747.7477477477, 949549.5495495495, 951351.3513513514, 953153.1531531531, 954954.9549549549, 956756.7567567567, 958558.5585585586, 960360.3603603604, 962162.1621621621, 963963.9639639639, 965765.7657657657, 967567.5675675676, 969369.3693693693, 971171.1711711711, 972972.9729729729, 974774.7747747748, 976576.5765765766, 978378.3783783783, 980180.1801801801, 981981.9819819819, 983783.7837837838, 985585.5855855856, 987387.3873873873, 989189.1891891891, 990990.990990991, 992792.7927927928, 994594.5945945946, 996396.3963963963, 998198.1981981982, 1000000.0, 1001801.8018018018, 1003603.6036036036, 1005405.4054054053, 1007207.2072072072, 1009009.009009009, 1010810.8108108108, 1012612.6126126125, 1014414.4144144144, 1016216.2162162162, 1018018.018018018, 1019819.8198198198, 1021621.6216216215, 1023423.4234234234, 1025225.2252252252, 1027027.027027027, 1028828.8288288288, 1030630.6306306307, 1032432.4324324324, 1034234.2342342342, 1036036.036036036, 1037837.8378378378, 1039639.6396396396, 1041441.4414414414, 1043243.2432432432, 1045045.045045045, 1046846.8468468469, 1048648.6486486485, 1050450.4504504504, 1052252.2522522523, 1054054.054054054, 1055855.8558558559, 1057657.6576576577, 1059459.4594594594, 1061261.261261261, 1063063.0630630632, 1064864.8648648649, 1066666.6666666665, 1068468.4684684684, 1070270.2702702703, 1072072.072072072, 1073873.8738738738, 1075675.6756756757, 1077477.4774774774, 1079279.2792792793, 1081081.0810810812, 1082882.8828828828, 1084684.6846846845, 1086486.4864864866, 1088288.2882882883, 1090090.09009009, 1091891.8918918918, 1093693.6936936937, 1095495.4954954954, 1097297.2972972973, 1099099.0990990992, 1100900.9009009008, 1102702.7027027027, 1104504.5045045046, 1106306.3063063063, 1108108.108108108, 1109909.9099099098, 1111711.7117117117, 1113513.5135135134, 1115315.3153153153, 1117117.1171171172, 1118918.9189189188, 1120720.7207207207, 1122522.5225225226, 1124324.3243243243, 1126126.126126126, 1127927.927927928, 1129729.7297297297, 1131531.5315315314, 1133333.3333333333, 1135135.1351351351, 1136936.9369369368, 1138738.7387387387, 1140540.5405405406, 1142342.3423423423, 1144144.1441441441, 1145945.945945946, 1147747.7477477477, 1149549.5495495494, 1151351.3513513515, 1153153.1531531531, 1154954.9549549548, 1156756.7567567567, 1158558.5585585586, 1160360.3603603602, 1162162.1621621621, 1163963.963963964, 1165765.7657657657, 1167567.5675675676, 1169369.3693693695, 1171171.1711711711, 1172972.9729729728, 1174774.774774775, 1176576.5765765766, 1178378.3783783782, 1180180.1801801801, 1181981.981981982, 1183783.7837837837, 1185585.5855855856, 1187387.3873873875, 1189189.189189189, 1190990.990990991, 1192792.792792793, 1194594.5945945946, 1196396.3963963962, 1198198.198198198, 1200000.0, 1201801.8018018017, 1203603.6036036036, 1205405.4054054054, 1207207.207207207, 1209009.009009009, 1210810.810810811, 1212612.6126126125, 1214414.4144144142, 1216216.2162162163, 1218018.018018018, 1219819.8198198196, 1221621.6216216215, 1223423.4234234234, 1225225.225225225, 1227027.027027027, 1228828.8288288289, 1230630.6306306305, 1232432.4324324324, 1234234.2342342343, 1236036.036036036, 1237837.8378378376, 1239639.6396396398, 1241441.4414414414, 1243243.243243243, 1245045.045045045, 1246846.8468468469, 1248648.6486486485, 1250450.4504504504, 1252252.2522522523, 1254054.054054054, 1255855.8558558559, 1257657.6576576575, 1259459.4594594594, 1261261.2612612613, 1263063.063063063, 1264864.8648648649, 1266666.6666666665, 1268468.4684684684, 1270270.2702702703, 1272072.072072072, 1273873.8738738738, 1275675.6756756757, 1277477.4774774774, 1279279.2792792793, 1281081.081081081, 1282882.8828828828, 1284684.6846846847, 1286486.4864864864, 1288288.2882882883, 1290090.09009009, 1291891.8918918918, 1293693.6936936937, 1295495.4954954954, 1297297.2972972973, 1299099.0990990992, 1300900.9009009008, 1302702.7027027027, 1304504.5045045044, 1306306.3063063063, 1308108.1081081082, 1309909.9099099098, 1311711.7117117117, 1313513.5135135134, 1315315.3153153153, 1317117.1171171172, 1318918.9189189188, 1320720.7207207207, 1322522.5225225224, 1324324.3243243243, 1326126.1261261262, 1327927.9279279278, 1329729.7297297297, 1331531.5315315316, 1333333.3333333333, 1335135.1351351351, 1336936.9369369368, 1338738.7387387387, 1340540.5405405406, 1342342.3423423423, 1344144.1441441441, 1345945.9459459458, 1347747.7477477477, 1349549.5495495496, 1351351.3513513512, 1353153.1531531531, 1354954.9549549548, 1356756.7567567567, 1358558.5585585586, 1360360.3603603602, 1362162.1621621621, 1363963.963963964, 1365765.7657657657, 1367567.5675675676, 1369369.3693693692, 1371171.1711711711, 1372972.972972973, 1374774.7747747747, 1376576.5765765766, 1378378.3783783782, 1380180.1801801801, 1381981.981981982, 1383783.7837837837, 1385585.5855855856, 1387387.3873873875, 1389189.189189189, 1390990.990990991, 1392792.7927927927, 1394594.5945945946, 1396396.3963963964, 1398198.198198198, 1400000.0, 1401801.8018018017, 1403603.6036036036, 1405405.4054054054, 1407207.207207207, 1409009.009009009, 1410810.8108108107, 1412612.6126126125, 1414414.4144144144, 1416216.216216216, 1418018.018018018, 1419819.8198198199, 1421621.6216216215, 1423423.4234234234, 1425225.225225225, 1427027.027027027, 1428828.8288288289, 1430630.6306306305, 1432432.4324324324, 1434234.234234234, 1436036.036036036, 1437837.8378378379, 1439639.6396396395, 1441441.4414414414, 1443243.243243243, 1445045.045045045, 1446846.8468468469, 1448648.6486486485, 1450450.4504504504, 1452252.2522522523, 1454054.054054054, 1455855.8558558559, 1457657.6576576575, 1459459.4594594594, 1461261.2612612613, 1463063.063063063, 1464864.8648648649, 1466666.6666666665, 1468468.4684684684, 1470270.2702702703, 1472072.072072072, 1473873.8738738738, 1475675.6756756757, 1477477.4774774774, 1479279.2792792793, 1481081.081081081, 1482882.8828828828, 1484684.6846846847, 1486486.4864864864, 1488288.2882882883, 1490090.09009009, 1491891.8918918918, 1493693.6936936937, 1495495.4954954954, 1497297.2972972973, 1499099.099099099, 1500900.9009009008, 1502702.7027027027, 1504504.5045045044, 1506306.3063063063, 1508108.1081081082, 1509909.9099099098, 1511711.7117117117, 1513513.5135135134, 1515315.3153153153, 1517117.1171171172, 1518918.9189189188, 1520720.7207207207, 1522522.5225225224, 1524324.3243243243, 1526126.1261261262, 1527927.9279279278, 1529729.7297297297, 1531531.5315315314, 1533333.3333333333, 1535135.1351351351, 1536936.9369369368, 1538738.7387387387, 1540540.5405405406, 1542342.3423423423, 1544144.1441441441, 1545945.9459459458, 1547747.7477477477, 1549549.5495495496, 1551351.3513513512, 1553153.1531531531, 1554954.9549549548, 1556756.7567567567, 1558558.5585585586, 1560360.3603603602, 1562162.1621621621, 1563963.963963964, 1565765.7657657657, 1567567.5675675676, 1569369.3693693692, 1571171.1711711711, 1572972.972972973, 1574774.7747747747, 1576576.5765765766, 1578378.3783783782, 1580180.1801801801, 1581981.981981982, 1583783.7837837837, 1585585.5855855856, 1587387.3873873872, 1589189.189189189, 1590990.990990991, 1592792.7927927927, 1594594.5945945946, 1596396.3963963964, 1598198.198198198, 1600000.0, 1601801.8018018017, 1603603.6036036036, 1605405.4054054054, 1607207.207207207, 1609009.009009009, 1610810.8108108107, 1612612.6126126125, 1614414.4144144144, 1616216.216216216, 1618018.018018018, 1619819.8198198196, 1621621.6216216215, 1623423.4234234234, 1625225.225225225, 1627027.027027027, 1628828.8288288289, 1630630.6306306305, 1632432.4324324324, 1634234.234234234, 1636036.036036036, 1637837.8378378379, 1639639.6396396395, 1641441.4414414414, 1643243.243243243, 1645045.045045045, 1646846.8468468469, 1648648.6486486485, 1650450.4504504504, 1652252.2522522523, 1654054.054054054, 1655855.8558558559, 1657657.6576576575, 1659459.4594594594, 1661261.2612612613, 1663063.063063063, 1664864.8648648649, 1666666.6666666665, 1668468.4684684684, 1670270.2702702703, 1672072.072072072, 1673873.8738738738, 1675675.6756756755, 1677477.4774774774, 1679279.2792792793, 1681081.081081081, 1682882.8828828828, 1684684.6846846847, 1686486.4864864864, 1688288.2882882883, 1690090.09009009, 1691891.8918918918, 1693693.6936936937, 1695495.4954954954, 1697297.2972972973, 1699099.099099099, 1700900.9009009008, 1702702.7027027027, 1704504.5045045044, 1706306.3063063063, 1708108.108108108, 1709909.9099099098, 1711711.7117117117, 1713513.5135135134, 1715315.3153153153, 1717117.1171171172, 1718918.9189189188, 1720720.7207207207, 1722522.5225225224, 1724324.3243243243, 1726126.1261261262, 1727927.9279279278, 1729729.7297297297, 1731531.5315315314, 1733333.3333333333, 1735135.1351351351, 1736936.9369369368, 1738738.7387387387, 1740540.5405405406, 1742342.3423423423, 1744144.1441441441, 1745945.9459459458, 1747747.7477477477, 1749549.5495495496, 1751351.3513513512, 1753153.1531531531, 1754954.9549549548, 1756756.7567567567, 1758558.5585585586, 1760360.3603603602, 1762162.1621621621, 1763963.9639639638, 1765765.7657657657, 1767567.5675675676, 1769369.3693693692, 1771171.1711711711, 1772972.972972973, 1774774.7747747747, 1776576.5765765766, 1778378.3783783782, 1780180.1801801801, 1781981.981981982, 1783783.7837837837, 1785585.5855855856, 1787387.3873873872, 1789189.189189189, 1790990.990990991, 1792792.7927927927, 1794594.5945945946, 1796396.3963963964, 1798198.198198198, 1800000.0, 1801801.8018018017, 1803603.6036036036, 1805405.4054054054, 1807207.207207207, 1809009.009009009, 1810810.8108108107, 1812612.6126126125, 1814414.4144144144, 1816216.216216216, 1818018.018018018, 1819819.8198198196, 1821621.6216216215, 1823423.4234234234, 1825225.225225225, 1827027.027027027, 1828828.8288288289, 1830630.6306306305, 1832432.4324324324, 1834234.234234234, 1836036.036036036, 1837837.8378378379, 1839639.6396396395, 1841441.4414414414, 1843243.243243243, 1845045.045045045, 1846846.8468468469, 1848648.6486486485, 1850450.4504504504, 1852252.252252252, 1854054.054054054, 1855855.8558558559, 1857657.6576576575, 1859459.4594594594, 1861261.2612612613, 1863063.063063063, 1864864.8648648649, 1866666.6666666665, 1868468.4684684684, 1870270.2702702703, 1872072.072072072, 1873873.8738738738, 1875675.6756756755, 1877477.4774774774, 1879279.2792792793, 1881081.081081081, 1882882.8828828828, 1884684.6846846847, 1886486.4864864864, 1888288.2882882883, 1890090.09009009, 1891891.8918918918, 1893693.6936936937, 1895495.4954954954, 1897297.2972972973, 1899099.099099099, 1900900.9009009008, 1902702.7027027027, 1904504.5045045044, 1906306.3063063063, 1908108.108108108, 1909909.9099099098, 1911711.7117117117, 1913513.5135135134, 1915315.3153153153, 1917117.1171171172, 1918918.9189189188, 1920720.7207207207, 1922522.5225225224, 1924324.3243243243, 1926126.1261261262, 1927927.9279279278, 1929729.7297297297, 1931531.5315315314, 1933333.3333333333, 1935135.1351351351, 1936936.9369369368, 1938738.7387387387, 1940540.5405405404, 1942342.3423423423, 1944144.1441441441, 1945945.9459459458, 1947747.7477477477, 1949549.5495495496, 1951351.3513513512, 1953153.1531531531, 1954954.9549549548, 1956756.7567567567, 1958558.5585585586, 1960360.3603603602, 1962162.1621621621, 1963963.9639639638, 1965765.7657657657, 1967567.5675675676, 1969369.3693693692, 1971171.1711711711, 1972972.972972973, 1974774.7747747747, 1976576.5765765766, 1978378.3783783782, 1980180.1801801801, 1981981.981981982, 1983783.7837837837, 1985585.5855855856, 1987387.3873873872, 1989189.189189189, 1990990.990990991, 1992792.7927927927, 1994594.5945945946, 1996396.3963963962, 1998198.198198198, 2000000.0] ("RAW Freq table")) -> ()
      n12 = local read "VNA Settings cluster"() -> (w32:T10)
      n13 = Divide(x=w27, y=w26) -> (x/y=w25:dbl)
      n14 = Divide(x=w42, y=w43) -> (x/y=w29:dbl)
      n15 = Divide(x=w41, y=w43) -> (x/y=w30:dbl)
      n16 = Bundle By Name(cluster=w45, "F start"=w42, "F stop"=w41, "Sweep size"=w26, "Decimation"=u32 1000, "F_corr"=u32 0, "Ph_OUT1"=u32 0, "Ph_OUT2"=u32 0 ("F_corr"), "OUT_Lvl1"=u32 32700 ("F_corr"), "OUT_Lvl2"=u32 0 ("F_corr"), "GPIO"=u32 0 ("F_corr")) -> (w44:T1)
      n17 = local write "START"(w29) -> ()
      n18 = local write "STOP"(w30) -> ()
      n19 = local write "RP VNA SETTING"(w44) -> ()
      n20 = local write "CENTER"(w28) -> ()
      n21 = Bundle By Name(cluster=w32, "START 2"=w29, "STOP 2"=w30, "CENTER 2"=w28, "SPAN 2"=w27, "PUMP"=w24, "PROBE"=w24, "Points N° 2"=w26, "SPACING 2"=w25) -> (w31:T10)
      n22 = local write "VNA Settings cluster"(w31) -> ()
      n23 = invoke on="VNA DATA CLUSTER TBL" class="Arr (strict)" method="Reinit To Default"() -> ()  [unwired: 3 in, 3 out]
      n24 = local write "CHANNELS PARAMETERS"(T4 [{"START 2"=200.0, "STOP 2"=2000.5, "CENTER 2"=1050.0, "SPAN 2"=1800.0, "CHANNEL TRACK ?"=FALSE, "PUMP"=100.0, "PROBE"=100.0, "Points N° 2"=1000, "SPACING 2"=100.0, "Parafit span"=500.0, "Parafit span type"=enum."Points N°"}, {"START 2"=200.0, "STOP 2"=2000.0, "CENTER 2"=1100.0, "SPAN 2"=1800.0, "CHANNEL TRACK ?"=FALSE, "PUMP"=100.0, "PROBE"=100.0, "Points N° 2"=1000, "SPACING 2"=1800.0, "Parafit span"=0.0, "Parafit span type"=enum."Points N°"}, {"START 2"=200.0, "STOP 2"=2000.0, "CENTER 2"=1100.0, "SPAN 2"=1800.0, "CHANNEL TRACK ?"=FALSE, "PUMP"=100.0, "PROBE"=100.0, "Points N° 2"=1000, "SPACING 2"=1800.0, "Parafit span"=0.0, "Parafit span type"=enum."Points N°"}, {"START 2"=200.0, "STOP 2"=2000.0, "CENTER 2"=1100.0, "SPAN 2"=1800.0, "CHANNEL TRACK ?"=FALSE, "PUMP"=100.0, "PROBE"=100.0, "Points N° 2"=1000, "SPACING 2"=1800.0, "Parafit span"=0.0, "Parafit span type"=enum."Points N°"}, {"START 2"=200.0, "STOP 2"=2000.0, "CENTER 2"=1100.0, "SPAN 2"=1800.0, "CHANNEL TRACK ?"=FALSE, "PUMP"=100.0, "PROBE"=100.0, "Points N° 2"=1000, "SPACING 2"=1800.0, "Parafit span"=0.0, "Parafit span type"=enum."Points N°"}, {"START 2"=200.0, "STOP 2"=2000.0, "CENTER 2"=1100.0, "SPAN 2"=1800.0, "CHANNEL TRACK ?"=FALSE, "PUMP"=100.0, "PROBE"=100.0, "Points N° 2"=1000, "SPACING 2"=1800.0, "Parafit span"=0.0, "Parafit span type"=enum."Points N°"}, {"START 2"=200.0, "STOP 2"=2000.0, "CENTER 2"=1100.0, "SPAN 2"=1800.0, "CHANNEL TRACK ?"=FALSE, "PUMP"=100.0, "PROBE"=100.0, "Points N° 2"=1000, "SPACING 2"=1800.0, "Parafit span"=0.0, "Parafit span type"=enum."Points N°"}, {"START 2"=200.0, "STOP 2"=2000.0, "CENTER 2"=1100.0, "SPAN 2"=1800.0, "CHANNEL TRACK ?"=FALSE, "PUMP"=100.0, "PROBE"=100.0, "Points N° 2"=1000, "SPACING 2"=1800.0, "Parafit span"=0.0, "Parafit span type"=enum."Points N°"}, {"START 2"=200.0, "STOP 2"=2000.0, "CENTER 2"=1100.0, "SPAN 2"=1800.0, "CHANNEL TRACK ?"=FALSE, "PUMP"=100.0, "PROBE"=100.0, "Points N° 2"=1000, "SPACING 2"=1800.0, "Parafit span"=0.0, "Parafit span type"=enum."Points N°"}, {"START 2"=200.0, "STOP 2"=2000.0, "CENTER 2"=1100.0, "SPAN 2"=1800.0, "CHANNEL TRACK ?"=FALSE, "PUMP"=100.0, "PROBE"=100.0, "Points N° 2"=1000, "SPACING 2"=1800.0, "Parafit span"=0.0, "Parafit span type"=enum."Points N°"}, {"START 2"=200.0, "STOP 2"=2000.0, "CENTER 2"=1100.0, "SPAN 2"=1800.0, "CHANNEL TRACK ?"=FALSE, "PUMP"=100.0, "PROBE"=100.0, "Points N° 2"=1000, "SPACING 2"=1800.0, "Parafit span"=0.0, "Parafit span type"=enum."Points N°"}, {"START 2"=200.0, "STOP 2"=2000.0, "CENTER 2"=1100.0, "SPAN 2"=1800.0, "CHANNEL TRACK ?"=FALSE, "PUMP"=100.0, "PROBE"=100.0, "Points N° 2"=1000, "SPACING 2"=1800.0, "Parafit span"=0.0, "Parafit span type"=enum."Points N°"}, {"START 2"=200.0, "STOP 2"=2000.0, "CENTER 2"=1100.0, "SPAN 2"=1800.0, "CHANNEL TRACK ?"=FALSE, "PUMP"=100.0, "PROBE"=100.0, "Points N° 2"=1000, "SPACING 2"=1800.0, "Parafit span"=0.0, "Parafit span type"=enum."Points N°"}, {"START 2"=200.0, "STOP 2"=2000.0, "CENTER 2"=1100.0, "SPAN 2"=1800.0, "CHANNEL TRACK ?"=FALSE, "PUMP"=100.0, "PROBE"=100.0, "Points N° 2"=1000, "SPACING 2"=1800.0, "Parafit span"=0.0, "Parafit span type"=enum."Points N°"}, {"START 2"=200.0, "STOP 2"=2000.0, "CENTER 2"=1100.0, "SPAN 2"=1800.0, "CHANNEL TRACK ?"=FALSE, "PUMP"=100.0, "PROBE"=100.0, "Points N° 2"=1000, "SPACING 2"=1800.0, "Parafit span"=0.0, "Parafit span type"=enum."Points N°"}, {"START 2"=200.0, "STOP 2"=2000.0, "CENTER 2"=1100.0, "SPAN 2"=1800.0, "CHANNEL TRACK ?"=FALSE, "PUMP"=100.0, "PROBE"=100.0, "Points N° 2"=1000, "SPACING 2"=1800.0, "Parafit span"=0.0, "Parafit span type"=enum."Points N°"}] ("CHANNELS PARAMETERS")) -> ()
      n25 = local read "TRACK DATA PARAMETERS"() -> (w19:cluster{"MAIN FOLDER":path})
      n26 = local read "TRACK DATA PARAMETERS"() -> (w4:cluster{"MAIN FOLDER":path})
      n27 = Unbundle By Name(w19) -> ("MAIN FOLDER"=w18:path)
      n28 = Unbundle By Name(w4) -> ("MAIN FOLDER"=w5:path)
      n29 = Build Path(base path=w18, name or relative path=path "Configuration file/conf.ini") -> (appended path=w16:path)
      n30 = Build Path(base path=w5, name or relative path=path "VOA calibration/PUMP.txt") -> (appended path=w8:path)
      n31 = Build Path(base path=w5, name or relative path=path "VOA calibration/PROBE.txt") -> (appended path=w9:path)
      n32 = local read "NETWORK PARAMETERS"() -> (w15:T7)
      n33 = call "RP - READ MAC CONF FILE.vi"("Path"=w16) -> ("RP2 MAC"=w13:string, "RP1 MAC"=w14:string)  [unwired: 8 in, 1 out]
      n34 = call "RP-VOA CALIBRATION FIT.vi"("file path"=w8) -> ("Calibration array"=w10:dbl[])  [unwired: 2 in, 1 out]
      n35 = call "RP-VOA CALIBRATION FIT.vi"("file path"=w9) -> ("Calibration array"=w11:dbl[])  [unwired: 2 in, 1 out]
      n36 = local read "VOA Calibration cluster"() -> (w6:cluster{"PUMP":dbl[], "PROBE":dbl[]})
      n37 = Bundle By Name(cluster=w15, "RP-MAC 1"=w14, "RP-MAC 2"=w13) -> (w12:T7)
      n38 = Bundle By Name(cluster=w6, "PUMP"=w10, "PROBE"=w11) -> (w7:cluster{"PUMP":dbl[], "PROBE":dbl[]})
      n39 = local write "NETWORK PARAMETERS"(w12) -> ()
      n40 = local write "VOA Calibration cluster"(w7) -> ()
    }
    frame #2 {
      # "CONNEXION WAIT"
      n41 = local read "NETWORK PARAMETERS"() -> (w51:T7)
      n42 = Unbundle By Name(w51) -> ("RP-MAC 1"=w50:string, "RP-MAC 2"=w49:string)
      n43 = call "RP-GET IP ADDRESS.vi"("MAC address"=w50) -> ("IP address"=w56:string)
      n44 = call "RP-GET IP ADDRESS.vi"("MAC address"=w49) -> ("IP address"=w53:string)
      n45 = local read "ENABLE INTERNAL MODULATION"() -> (w47:bool)
      n46 = Bundle By Name(cluster=w51, "RP-IP 1"=w56, "RP-IP 2"=w53) -> (w60:T7)
      n47 = String Length(string=w56) -> (length=w58:i32)
      n48 = String Length(string=w53) -> (length=w59:i32)
      n49 = call "VNARP - LAUNCH.vi"("RP IP"=w56) -> ("VNA launched ?"=w57:bool)  [unwired: 10 in]
      n50 = call "RP-START SCPI.vi"("RP IP"=w53) -> ("SCPI launched ?"=w52:bool)  [unwired: 10 in]
      n51 = Greater Than 0?(x=w58) -> (x > 0?=w55:bool)
      n52 = Greater Than 0?(x=w59) -> (x > 0?=w54:bool)
      n53 = local write "NETWORK PARAMETERS"(w60) -> ()
      n54 = Compound Arithmetic op=AND(w55, w54, w57, w52) -> (w46:bool)
      n55 = And(x=w46, y=w47) -> (x .and. y?=w48:bool)
      n56 = local write "RP CONNECT"(w46) -> ()
      n57 = case shown="True" w48 {
        frame False {
        }
        frame True {
          w63 = u16 1 items=["Channel 1"=1, "Channel 2"=2] ("Channel (1|2)")
          n58 = local read "NETWORK PARAMETERS"() -> (w62:T7)
          n59 = Unbundle By Name(w62) -> ("RP-IP 2"=w61:string)
          n60 = call "RP-GEN SINUS-OUT.vi"("Amplitude(1V)"="Amplitude(1V)", "Frequency (Hz)"=10000000, "Channel (1|2)"=w63, "IP address"=w61) -> ()  [unwired: 1 out]
        }
      }
    }
    frame #3 {
      w79 = ""  # données (peuvent avoir n'importe quel type)
      # "attente libération des deux piles avant fermeture"
      # "MAIN"
      n61 = local read "NETWORK PARAMETERS"() -> (w68:T7)
      n62 = local read "RP VNA SETTING"() -> (w75:T1)
      n63 = Unbundle By Name(w68) -> ("RP-IP 1"=w67:string)
      n64 = call "VNARP-Connexion.vi"("IP RP"=w67) -> ("sortie d'erreur"=w77:errorcluster, "ID de connexion"=w76:refnum<k5>)  [unwired: 1 in]
      n65 = Obtain Queue(element data type=w79) -> (queue out=w78:refnum<queue>, error out=w81:errorcluster)  [unwired: 4 in, 1 out]
      n66 = call "VNARP-SettingsUpdate.vi"("Error IN"=w77, "RP VNA SETTINGS IN"=w75, "ID de connexion IN"=w76) -> ("Error OUT"=w72:errorcluster, "Freq table"=w73:dbl[], "ID de connexion OUT"=w74:refnum<k5>)
      n67 = while {
        shift-right: [w610] -> w80
        shift-left: w81 -> [w612]
        tunnel: w78 -> [w613]
        tunnel: [w608] -> w71
        stop <- w608 stop-if-true
        n68 = event shown="[24] \"BTN VIEW PERSISTANCE\": Mouse Up" {
          selector: _ -> [_ _ _ _ _ _ _ _ _ _ _ _ _ _ _ _ _ _ _ _ _ _ _ _ _]
          dyn-events: _ -> [_ _ _ _ _ _ _ _ _ _ _ _ _ _ _ _ _ _ _ _ _ _ _ _ _]
          timeout: 250 -> [_ _ _ _ _ _ _ _ _ _ _ _ _ _ _ _ _ _ _ _ _ _ _ _ _]
          tunnel: w613 -> [w618 w621 w625 _ _ w643 _ w668 w690 w716 w742 w765 w777 w806 _ _ _ _ _ w819 _ w845 _ w853 _]
          tunnel: w612 -> [w616 w620 w624 _ _ w642 _ w667 w689 w715 w744 w764 w776 w805 _ _ _ _ _ w818 _ w846 _ w852 _]
          tunnel: [w615 w619 w623 _ _ w641 _ w666 w688 w713 w743 w763 w775 w807 _ _ _ _ _ w817 _ w844 _ w851 _] -> w610
          tunnel: [_ _ _ _ _ _ _ _ _ _ _ _ _ w803 _ _ _ _ _ _ _ _ _ _ _] -> w611
          event "BTN LOOP VNA": Value Change {
            n69 = event-data() -> ("NewVal"=w614:bool)  [unwired: 1 in]
            n70 = local write "LOOP ACT"(w614) -> ()
            n71 = Enqueue Element(queue=w618, element="VNA LOOP", error in (no error)=w616) -> (error out=w615:errorcluster)  [unwired: 1 in, 2 out]
          }
          event "BTN RUN VNA": Value Change {
            n72 = event-data() -> ()  [unwired: 1 in, 2 out]
            n73 = Enqueue Element(queue=w621, element="RUN VNA", error in (no error)=w620) -> (error out=w619:errorcluster)  [unwired: 1 in, 2 out]
          }
          event "PUMP", "PROBE": Mouse Up {
            n74 = event-data() -> ()  [unwired: 1 in, 2 out]
            n75 = Enqueue Element(queue=w625, element="POWER UPDATE", error in (no error)=w624) -> (error out=w623:errorcluster)  [unwired: 1 in, 2 out]
          }
          event "Hide/Show track data channel": Value Change {
            # "TO TEST ON ALPHA"
            n76 = event-data() -> ()  [unwired: 1 in, 2 out]
            n77 = local read "Hide/Show track data channel"() -> (w627:bool[])
            n78 = for {
              tunnel: w627 -> [w628] mode=indexing
              i -> [w629]
              n79 = flat-sequence {
                tunnel: w629 -> [w630]
                tunnel: w628 -> [w631]
                frame #0 {
                  n80 = property on="LIVE TRACK" class="WFGraph (strict)"("Active Plot"=w630) -> ()  [unwired: 2 in, 2 out]
                }
                frame #1 {
                  n81 = property on="LIVE TRACK" class="WFGraph (strict)"("Plot.Visible?"=w631) -> ()  [unwired: 2 in, 2 out]
                }
              }
            }
          }
          event "MAGNITUDE/PHASE": Value Change {
            n82 = event-data() -> ()  [unwired: 1 in, 2 out]
            n83 = local read "Autoscale"() -> (w632:bool)
            n84 = case shown="True" w632 {
              frame False {
              }
              frame True {
                n85 = flat-sequence {
                  frame #0 {
                    n86 = property on="MAGNITUDE/PHASE" class="XYGraph (strict)"("ActYScl"=0 ("Active Y Scale")) -> ()  [unwired: 2 in, 2 out]
                  }
                  frame #1 {
                    n87 = local read "VNA DATA CLUSTER"() -> (w637:T8)
                    n88 = Unbundle By Name(w637) -> ("MAGNITUDE TABLE"=w638:ext[])
                    n89 = Array Max & Min(array=w638) -> (max value=w639:ext)  [unwired: 3 out]
                    n90 = Multiply(x=1.1, y=w639) -> (x*y=w635:ext)
                    n91 = property on="MAGNITUDE/PHASE" class="XYGraph (strict)"("YScale.Maximum"=w635, "YScale.Minimum"=0.0) -> ()  [unwired: 2 in, 2 out]
                  }
                }
              }
            }
          }
          event "CHANNEL CHOICE VNA": Value Change {
            n92 = event-data() -> ()  [unwired: 1 in, 2 out]
            n93 = Enqueue Element(queue=w643, element="CHANNEL CHANGE", error in (no error)=w642) -> (error out=w641:errorcluster)  [unwired: 1 in, 2 out]
            n94 = One Button Dialog(message="TRIGGERED !") -> ()  [unwired: 1 in, 1 out]
          }
          event "BTN NEW TRACK": Mouse Up {
            n95 = event-data() -> ()  [unwired: 1 in, 2 out]
            n96 = Two Button Dialog(message="Initiate a new tracking session ?") -> (T button?=w645:bool)  [unwired: 2 in]
            n97 = case shown="True" w645 {
              frame False {
              }
              frame True {
                n98 = stacked-sequence {
                  frame #0 {
                    # "LOCK ALL CONTROLS"
                  }
                  frame #1 {
                    n99 = local read "ASSAY NAME"() -> (w652:string)
                    n100 = local read "CHANNELS PARAMETERS"() -> (w653:T4)
                    n101 = local read "TRACK DATA PARAMETERS"() -> (w651:cluster{"MAIN FOLDER":path})
                    n102 = Unbundle By Name(w651) -> ("MAIN FOLDER"=w650:path)
                    n103 = call "RP-TRACKDataStructBuild.vi"("CHANNELS PARAMETERS"=w653, "Track session name"=w652, "SensWay track data path"=w650) -> ("TRACK REPOSITERY"=w649:path, "Track File List"=w648:path[], "Track Repositery List"=w647:path[])
                    n104 = local write "Track Repositery List"(w647) -> ()
                    n105 = local write "Track File List"(w648) -> ()
                    n106 = local write "TRACK REPOSITERY"(w649) -> ()
                  }
                  frame #2 {
                    n107 = local read "CHANNELS PARAMETERS"() -> (w655:T4)
                    n108 = for {
                      tunnel: w655 -> [w665] mode=indexing
                      border: cluster{"CHANNEL":dbl, "KPI 1 TRACK":ext[]}[] [] -> [_]
                      i -> [w661]
                      n109 = Unbundle By Name(w665) -> ("CHANNEL TRACK ?"=w656:bool)
                      n110 = Select(t=dbl[] [0.0], s=w656, f=dbl[] []) -> (s? t:f=w659:dbl[])
                      n111 = Bundle By Name(cluster=cluster{"CHANNEL":dbl, "KPI 1 TRACK":ext[]} {"CHANNEL"=0.0, "KPI 1 TRACK"=[0.0]} ("TRACK DATA CLUSTER"), "CHANNEL"=w661, "KPI 1 TRACK"=w659) -> (w660:cluster{"CHANNEL":dbl, "KPI 1 TRACK":ext[]})
                      n112 = feedback #1() -> (w663:cluster{"CHANNEL":dbl, "KPI 1 TRACK":ext[]}[])
                      n113 = Build Array (concatenate)(w663, w660) -> (w664:cluster{"CHANNEL":dbl, "KPI 1 TRACK":ext[]}[])
                      n114 = feedback-in #1(w664) -> ()
                      n115 = local write "TRACK DATA CLUSTER TBL"(w664) -> ()
                    }
                  }
                  frame #3 {
                  }
                }
              }
            }
          }
          event "START", "STOP": Value Change {
            n116 = event-data() -> ()  [unwired: 1 in, 1 out]
            n117 = stacked-sequence {
              frame #0 {
                n118 = local read "STOP"() -> (w674:dbl)
                n119 = local read "START"() -> (w673:dbl)
                n120 = Subtract(x=w674, y=w673) -> (x-y=w675:dbl)
                n121 = Add(x=w674, y=w673) -> (x+y=w672:dbl)
                n122 = local write "SPAN"(w675) -> ()
                n123 = Divide(x=w672, y=2.0) -> (x/y=w670:dbl)
                n124 = local write "CENTER"(w670) -> ()
              }
              frame #1 {
                n125 = local read "Points N°"() -> (w680:i32)
                n126 = local read "SPAN"() -> (w679:dbl)
                n127 = Divide(x=w679, y=w680) -> (x/y=w678:dbl)
                n128 = Multiply(x=w678, y=1000.0) -> (x*y=w677:dbl)
                n129 = local write "SPACING"(w677) -> ()
              }
              frame #2 {
                w681 = 1000
                n130 = local read "STOP"() -> (w683:dbl)
                n131 = local read "START"() -> (w685:dbl)
                n132 = Multiply(x=w685, y=w681) -> (x*y=w684:dbl)
                n133 = Multiply(x=w681, y=w683) -> (x*y=w682:dbl)
                n134 = local read "RP VNA SETTING"() -> (w687:T1)
                n135 = Bundle By Name(cluster=w687, "F start"=w684, "F stop"=w682) -> (w686:T1)
                n136 = local write "RP VNA SETTING"(w686) -> ()
              }
            }
            n137 = Enqueue Element(queue=w668, element="UPDATE", error in (no error)=w667) -> (error out=w666:errorcluster)  [unwired: 1 in, 2 out]
          }
          event "CENTER", "SPAN": Value Change {
            n138 = event-data() -> ()  [unwired: 1 in, 1 out]
            n139 = stacked-sequence {
              frame #0 {
                w693 = 100.0 ("y")
                n140 = local read "CENTER"() -> (w697:dbl)
                n141 = local read "SPAN"() -> (w699:dbl)
                n142 = Divide(x=w699, y=2.0) -> (x/y=w696:dbl)
                n143 = Subtract(x=w697, y=w696) -> (x-y=w694:dbl)
                n144 = Add(x=w697, y=w696) -> (x+y=w700:dbl)
                n145 = local write "STOP"(w700) -> ()
                n146 = Greater Or Equal?(x=w694, y=w693) -> (x >= y?=w695:bool)
                n147 = Select(t=w694, s=w695, f=w693) -> (s? t:f=w692:dbl)
                n148 = local write "START"(w692) -> ()
              }
              frame #1 {
                n149 = local read "Points N°"() -> (w705:i32)
                n150 = local read "SPAN"() -> (w704:dbl)
                n151 = Divide(x=w704, y=w705) -> (x/y=w703:dbl)
                n152 = Multiply(x=w703, y=1000.0) -> (x*y=w702:dbl)
                n153 = local write "SPACING"(w702) -> ()
              }
              frame #2 {
                w706 = 1000
                n154 = local read "STOP"() -> (w708:dbl)
                n155 = local read "START"() -> (w710:dbl)
                n156 = Multiply(x=w710, y=w706) -> (x*y=w709:dbl)
                n157 = Multiply(x=w706, y=w708) -> (x*y=w707:dbl)
                n158 = local read "RP VNA SETTING"() -> (w712:T1)
                n159 = Bundle By Name(cluster=w712, "F start"=w709, "F stop"=w707) -> (w711:T1)
                n160 = local write "RP VNA SETTING"(w711) -> ()
              }
            }
            n161 = Enqueue Element(queue=w690, element="UPDATE", error in (no error)=w689) -> (error out=w688:errorcluster)  [unwired: 1 in, 2 out]
          }
          event "BTN ZOOM+": Mouse Up; "BTN ZOOM+": Value Change {
            n162 = event-data() -> ()  [unwired: 1 in, 1 out]
            n163 = stacked-sequence {
              frame #0 {
                n164 = local read "SPAN"() -> (w719:dbl)
                n165 = Multiply(x=w719, y=0.8) -> (x*y=w717:dbl)
                n166 = local write "SPAN"(w717) -> ()
              }
              frame #1 {
                n167 = local read "Points N°"() -> (w724:i32)
                n168 = local read "SPAN"() -> (w723:dbl)
                n169 = Divide(x=w723, y=w724) -> (x/y=w722:dbl)
                n170 = Multiply(x=w722, y=1000.0) -> (x*y=w721:dbl)
                n171 = local write "SPACING"(w721) -> ()
              }
              frame #2 {
                w726 = 100.0 ("y")
                n172 = local read "SPAN"() -> (w729:dbl)
                n173 = local read "CENTER"() -> (w731:dbl)
                n174 = Divide(x=w729, y=2.0) -> (x/y=w730:dbl)
                n175 = Subtract(x=w731, y=w730) -> (x-y=w727:dbl)
                n176 = Add(x=w731, y=w730) -> (x+y=w733:dbl)
                n177 = local write "STOP"(w733) -> ()
                n178 = Greater Or Equal?(x=w727, y=w726) -> (x >= y?=w728:bool)
                n179 = Select(t=w727, s=w728, f=w726) -> (s? t:f=w725:dbl)
                n180 = local write "START"(w725) -> ()
              }
              frame #3 {
                w734 = 1000
                n181 = local read "STOP"() -> (w736:dbl)
                n182 = local read "START"() -> (w738:dbl)
                n183 = Multiply(x=w738, y=w734) -> (x*y=w737:dbl)
                n184 = Multiply(x=w734, y=w736) -> (x*y=w735:dbl)
                n185 = local read "RP VNA SETTING"() -> (w740:T1)
                n186 = Bundle By Name(cluster=w740, "F start"=w737, "F stop"=w735) -> (w739:T1)
                n187 = local write "RP VNA SETTING"(w739) -> ()
              }
            }
            n188 = Enqueue Element(queue=w716, element="UPDATE", error in (no error)=w715) -> (error out=w713:errorcluster)  [unwired: 1 in, 2 out]
          }
          event "BTN RESET VNA": Mouse Up {
            n189 = event-data() -> ()  [unwired: 1 in, 1 out]
            n190 = flat-sequence {
              tunnel: w742 -> [w746]
              tunnel: [w746] -> w741
              frame #0 {
                w755 = u32 1000 ("Decimation")
                w753 = u32 2000000 ("Decimation")
                w754 = u32 200000 ("Decimation")
                w748 = u32 32700 ("F_corr")
                n191 = local read "RP VNA SETTING"() -> (w758:T1)
                n192 = local read "Points N°"() -> (w756:i32)
                n193 = Bundle By Name(cluster=w758, "F start"=w754, "F stop"=w753, "Sweep size"=w756, "Decimation"=u32 5000, "F_corr"=u32 0, "Ph_OUT1"=u32 0, "Ph_OUT2"=u32 0 ("F_corr"), "OUT_Lvl1"=w748, "OUT_Lvl2"=w748, "GPIO"=u32 0 ("F_corr")) -> (w757:T1)
                n194 = local write "RP VNA SETTING"(w757) -> ()
                n195 = Divide(x=w753, y=w755) -> (x/y=w759:dbl)
                n196 = Divide(x=w754, y=w755) -> (x/y=w760:dbl)
                n197 = local write "CENTER"(1050.0 ("Center")) -> ()
                n198 = local write "SPAN"(1900.0 ("Center")) -> ()
                n199 = local write "START"(w760) -> ()
                n200 = local write "STOP"(w759) -> ()
              }
            }
            n201 = Enqueue Element(queue=w741, element="UPDATE", error in (no error)=w744) -> (error out=w743:errorcluster)  [unwired: 1 in, 2 out]
          }
          event "Points N°": Value Change {
            n202 = event-data() -> ()  [unwired: 1 in, 1 out]
            n203 = stacked-sequence {
              frame #0 {
                n204 = local read "Points N°"() -> (w771:i32)
                n205 = local read "SPAN"() -> (w770:dbl)
                n206 = Divide(x=w770, y=w771) -> (x/y=w769:dbl)
                n207 = Multiply(x=w769, y=1000.0) -> (x*y=w768:dbl)
                n208 = local write "SPACING"(w768) -> ()
              }
              frame #1 {
                n209 = local read "Points N°"() -> (w772:i32)
                n210 = local read "RP VNA SETTING"() -> (w774:T1)
                n211 = Bundle By Name(cluster=w774, "Sweep size"=w772) -> (w773:T1)
                n212 = local write "RP VNA SETTING"(w773) -> ()
              }
            }
            n213 = Enqueue Element(queue=w765, element="UPDATE", error in (no error)=w764) -> (error out=w763:errorcluster)  [unwired: 1 in, 2 out]
          }
          event "BTN ZOOM-": Mouse Up {
            n214 = event-data() -> ()  [unwired: 1 in, 1 out]
            n215 = stacked-sequence {
              frame #0 {
                n216 = local read "SPAN"() -> (w781:dbl)
                n217 = Multiply(x=w781, y=1.2) -> (x*y=w779:dbl)
                n218 = local write "SPAN"(w779) -> ()
              }
              frame #1 {
                n219 = local read "Points N°"() -> (w786:i32)
                n220 = local read "SPAN"() -> (w785:dbl)
                n221 = Divide(x=w785, y=w786) -> (x/y=w784:dbl)
                n222 = Multiply(x=w784, y=1000.0) -> (x*y=w783:dbl)
                n223 = local write "SPACING"(w783) -> ()
              }
              frame #2 {
                w789 = 100.0 ("y")
                n224 = local read "SPAN"() -> (w791:dbl)
                n225 = local read "CENTER"() -> (w794:dbl)
                n226 = Divide(x=w791, y=2.0) -> (x/y=w793:dbl)
                n227 = Subtract(x=w794, y=w793) -> (x-y=w787:dbl)
                n228 = Add(x=w794, y=w793) -> (x+y=w795:dbl)
                n229 = Greater Or Equal?(x=w787, y=w789) -> (x >= y?=w790:bool)
                n230 = Select(t=w787, s=w790, f=w789) -> (s? t:f=w788:dbl)
                n231 = local write "STOP"(w795) -> ()
                n232 = local write "START"(w788) -> ()
              }
              frame #3 {
                w796 = 1000
                n233 = local read "STOP"() -> (w798:dbl)
                n234 = local read "START"() -> (w800:dbl)
                n235 = Multiply(x=w800, y=w796) -> (x*y=w799:dbl)
                n236 = Multiply(x=w796, y=w798) -> (x*y=w797:dbl)
                n237 = local read "RP VNA SETTING"() -> (w802:T1)
                n238 = Bundle By Name(cluster=w802, "F start"=w799, "F stop"=w797) -> (w801:T1)
                n239 = local write "RP VNA SETTING"(w801) -> ()
              }
            }
            n240 = Enqueue Element(queue=w777, element="UPDATE", error in (no error)=w776) -> (error out=w775:errorcluster)  [unwired: 1 in, 2 out]
          }
          event "BTN STOP": Value Change {
            n241 = event-data() -> ()  [unwired: 1 in, 1 out]
            n242 = Two Button Dialog(message="Are you sure you want to exit ?") -> (T button?=w803:bool)  [unwired: 2 in]
            n243 = case shown="True" w803 {
              tunnel: [w808 w811] -> w807
              tunnel: w806 -> [_ w810]
              tunnel: w805 -> [w808 w809]
              frame False {
              }
              frame True {
                n244 = Enqueue Element(queue=w810, element="STOP", error in (no error)=w809) -> (error out=w811:errorcluster)  [unwired: 1 in, 2 out]
              }
            }
          }
          event "PANEL GENERAL SETTINGS": Value Change {
            n245 = event-data() -> ()  [unwired: 1 in, 2 out]
            n246 = local write "MAIN TAB"(enum32{"Page 1", "Page 4", "Page 2", "Page 3"}."Page 3" ("Tab Control")) -> ()
          }
          event Timeout {
            n247 = event-data() -> ()  [unwired: 1 in, 2 out]
          }
          event "PANEL TRACK SETTINGS": Value Change {
            n248 = event-data() -> ()  [unwired: 1 in, 2 out]
            n249 = local write "MAIN TAB"(enum32{"Page 1", "Page 4", "Page 2", "Page 3"}."Page 2" ("Tab Control")) -> ()
          }
          event "PANEL VNA": Value Change {
            n250 = event-data() -> ()  [unwired: 1 in, 2 out]
            n251 = local write "MAIN TAB"(enum32{"Page 1", "Page 4", "Page 2", "Page 3"}."Page 1" ("Tab Control")) -> ()
          }
          event "PANEL TRACKING": Value Change {
            n252 = event-data() -> ()  [unwired: 1 in, 2 out]
            n253 = local write "MAIN TAB"(enum32{"Page 1", "Page 4", "Page 2", "Page 3"}."Page 4" ("Tab Control")) -> ()
          }
          event "BTN Center to max": Mouse Up; "BTN Center to max": Value Change {
            n254 = event-data() -> ()  [unwired: 1 in, 2 out]
            n255 = stacked-sequence {
              frame #0 {
                # "ATTENTION ! CONFUSION  freq table"
                n256 = local read "VNA DATA CLUSTER"() -> (w824:T8)
                n257 = Unbundle By Name(w824) -> ("FREQUENCY TABLE"=w823:ext[], "MAGNITUDE TABLE"=w822:ext[])
                n258 = Array Max & Min(array=w822) -> (max index (indices)=w827:i32)  [unwired: 3 out]
                n259 = Index Array(array=w823, index=w827) -> (element=w826:ext)
                n260 = Divide(x=w826, y=1000.0) -> (x/y=w821:ext)
                n261 = local write "CENTER"(w821) -> ()
                n262 = property on="CENTER" class="DigNum (strict)"("Val(Sgnl)"=w821) -> ()  [unwired: 2 in, 2 out]
              }
              frame #1 {
                w830 = 1000
                n263 = local read "START"() -> (w828:dbl)
                n264 = local read "STOP"() -> (w829:dbl)
                n265 = Multiply(x=w828, y=w830) -> (x*y=w832:dbl)
                n266 = Multiply(x=w830, y=w829) -> (x*y=w831:dbl)
                n267 = local read "RP VNA SETTING"() -> (w834:T1)
                n268 = Bundle By Name(cluster=w834, "F start"=w832, "F stop"=w831) -> (w833:T1)
                n269 = local write "RP VNA SETTING"(w833) -> ()
              }
            }
            n270 = Enqueue Element(queue=w819, element="UPDATE", error in (no error)=w818) -> (error out=w817:errorcluster)  [unwired: 1 in, 2 out]
          }
          event "BTN AF VNA": Mouse Up {
            n271 = event-data() -> ()  [unwired: 1 in, 2 out]
            n272 = local read "AUTOFOCUS PARAMETERS"() -> (w836:cluster{"ITERATIONS":i32})
            n273 = Unbundle By Name(w836) -> ("ITERATIONS"=w835:i32)
            n274 = for {
              N: w835 -> [_]
              tunnel: [w839] -> w837
              n275 = flat-sequence {
                tunnel: [w840] -> w839
                frame #0 {
                  w840 = FALSE ("Valeur (Signalisation)")
                  n276 = property on="BTN Center to max" class="Bool (strict)"("Val(Sgnl)"=w840) -> ()  [unwired: 2 in, 2 out]
                }
                frame #1 {
                  n277 = property on="BTN ZOOM+" class="Bool (strict)"("Val(Sgnl)"=FALSE ("Valeur (Signalisation)")) -> ()  [unwired: 2 in, 2 out]
                }
              }
              n278 = Wait (ms)(milliseconds to wait=u32 250 ("attente (ms)")) -> ()  [unwired: 1 out]
            }
            n279 = property on="BTN Center to max" class="Bool (strict)"("Val(Sgnl)"=w837) -> ()  [unwired: 2 in, 2 out]
          }
          event "BTN RUN TRACK": Value Change {
            w842 = TRUE ("x")
            n280 = event-data() -> ()  [unwired: 1 in, 2 out]
            n281 = Not(x=w842) -> (.not. x?=w843:bool)
            n282 = local write "LOOP ACT"(w842) -> ()
            n283 = property on="BTN PAUSE TRACK" class="Bool (strict)"("Visible"=w842) -> ()  [unwired: 2 in, 2 out]
            n284 = Enqueue Element(queue=w845, element="TRACK", error in (no error)=w846) -> (error out=w844:errorcluster)  [unwired: 1 in, 2 out]
            n285 = property on="BTN RUN TRACK" class="Bool (strict)"("Visible"=w843) -> ()  [unwired: 2 in, 2 out]
          }
          event "BTN PAUSE TRACK": Mouse Up {
            w848 = FALSE ("x")
            n286 = event-data() -> ()  [unwired: 1 in, 2 out]
            n287 = Not(x=w848) -> (.not. x?=w849:bool)
            n288 = local write "LOOP ACT"(w848) -> ()
            n289 = property on="BTN PAUSE TRACK" class="Bool (strict)"("Visible"=w848) -> ()  [unwired: 2 in, 2 out]
            n290 = property on="BTN RUN TRACK" class="Bool (strict)"("Visible"=w849) -> ()  [unwired: 2 in, 2 out]
          }
          event "BTN SAVE VNA": Mouse Up {
            n291 = event-data() -> ()  [unwired: 1 in, 2 out]
            n292 = Enqueue Element(queue=w853, element="SAVE VNA", error in (no error)=w852) -> (error out=w851:errorcluster)  [unwired: 1 in, 2 out]
          }
          event "BTN VIEW PERSISTANCE": Mouse Up {
            n293 = event-data() -> ()  [unwired: 1 in, 2 out]
            n294 = local read "VNA DATA CLUSTER"() -> (w854:T8)
            n295 = local write "PERSISTANCE DATA CLUSTER"(w854) -> ()
          }
        }
        n296 = Or(x=w610, y=w611) -> (x .or. y?=w608:bool)
        n297 = Wait (ms)(milliseconds to wait=u32 50 ("attente (ms)")) -> ()  [unwired: 1 out]
      }
      n298 = while {
        tunnel: w78 -> [w90]
        tunnel: w74 -> [w88]
        tunnel: w73 -> [w87]
        tunnel: w72 -> [w86]
        tunnel: [w85] -> w70
        border: dbl[] [0.0] -> [_]
        stop <- w85 stop-if-true
        n299 = Dequeue Element(queue=w90) -> (queue out=w89:refnum<queue>, element=w91:string, error out=w92:errorcluster)  [unwired: 2 in, 1 out]
        n300 = case shown="No Error" w92 {
          selector: w92 -> [w97 _]
          tunnel: w91 -> [w99 _]
          tunnel: [w93 TRUE] -> w85
          tunnel: w89 -> [w98 _]
          tunnel: w88 -> [w96 _]
          tunnel: w87 -> [w95 _]
          tunnel: w86 -> [w94 _]
          frame No Error {
            n301 = case shown="\"TRACK\"" w99 {
              selector: w99 -> [w106 w155 w217 w446 _ w523 w528 w548 _ w599]
              tunnel: w98 -> [w104 w150 w213 _ _ _ _ _ _ _]
              tunnel: w97 -> [_ _ _ _ _ _ _ _ _ _]
              tunnel: w96 -> [w103 w152 w215 w444 _ _ w527 _ _ w602]
              tunnel: w95 -> [w102 _ _ _ _ _ _ _ _ _]
              tunnel: w94 -> [w101 w151 w214 w443 _ _ w526 _ _ w601]
              tunnel: [FALSE FALSE FALSE FALSE FALSE FALSE FALSE FALSE FALSE TRUE] -> w93
              frame "VNA LOOP", Default {
                n302 = local write "STATUS"(w106) -> ()
                n303 = stacked-sequence {
                  tunnel: w103 -> [w116 _ _]
                  tunnel: w102 -> [_ _ _]
                  tunnel: w101 -> [w115 _ _]
                  tunnel: w104 -> [_ _ w146]
                  frame #0 {
                    (unwired) 10 ("kernel size (pts)")
                    n304 = local read "SPECTRUM POST PROCESSING PARAMETERS"() -> (w111:cluster{"N° SMOOTHING POINTS":i32})
                    n305 = local read "RP VNA SETTING"() -> (w129:T1)
                    n306 = Unbundle By Name(w111) -> ("N° SMOOTHING POINTS"=w110:i32)
                    n307 = Unbundle By Name(w129) -> ("Sweep size"=w128:u32)
                    n308 = local read "RAW Freq table"() -> (w124:dbl[])
                    n309 = local read "VNA DATA CLUSTER"() -> (w114:T8)
                    n310 = call "VNARP-CASES.vi"("entrée d'erreur (pas d'erreur)"=w115, "Setting"=u32 0, "Énum"=T11."SWEEP START", "ID de connexion"=w116) -> ("sortie d'erreur"=w125:errorcluster, "ID de connexion en sortie"=w130:refnum<k5>)  [unwired: 3 in]
                    n311 = call "VNARP-Read.vi"("ID de connexion"=w130, "entrée d'erreur (pas d'erreur)"=w125, "SIZE"=w128) -> ("MAGNITUDE 1"=w127:sgl[], "PHASE 1"=w126:dbl[])  [unwired: 9 in, 6 out]
                    n312 = call "VNARP-BOXCAR.vi"("Y IN"=w127, "kernel size (pts)"=w110, "Freq table IN"=w124) -> ("Y OUT"=w108:dbl[], "Freq table OUT"=w123:dbl[])  [unwired: 1 in]
                    n313 = call "VNARP-BOXCAR.vi"("Y IN"=w126, "kernel size (pts)"=w110, "Freq table IN"=w124) -> ("Y OUT"=w107:dbl[], "Freq table OUT"=w112:dbl[])  [unwired: 1 in]
                    n314 = Bundle By Name(cluster=w114, "FREQUENCY TABLE"=w112, "MAGNITUDE TABLE"=w108, "PHASE TABLE"=w107) -> (w113:T8)
                    n315 = Build Cluster Array(w123, w108) -> (w121:cluster{dbl, dbl}[])
                    n316 = Build Cluster Array(w112, w107) -> (w122:cluster{dbl, dbl}[])
                    n317 = local write "VNA DATA CLUSTER"(w113) -> ()
                    n318 = Bundle(w121) -> (w120:cluster{cluster{dbl, dbl}[]})  [unwired: 1 in]
                    n319 = Bundle(w122) -> (w119:cluster{cluster{dbl, dbl}[]})  [unwired: 1 in]
                    n320 = Build Array(w120, w119) -> (w109:cluster{cluster{dbl, dbl}[]}[])
                    n321 = local write "MAGNITUDE/PHASE"(w109) -> ()
                    n322 = property on="MAGNITUDE/PHASE" class="XYGraph (strict)"("Val(Sgnl)"=w109) -> ()  [unwired: 2 in, 2 out]
                  }
                  frame #1 {
                    n323 = local read "BTN VIEW PERSISTANCE"() -> (w131:bool)
                    n324 = case shown="True" w131 {
                      frame False {
                      }
                      frame True {
                        n325 = local read "PERSISTANCE DATA CLUSTER"() -> (w132:T8)
                        n326 = Unbundle By Name(w132) -> ("FREQUENCY TABLE"=w138:ext[], "MAGNITUDE TABLE"=w137:ext[], "PHASE TABLE"=w136:ext[])
                        n327 = Build Cluster Array(w138, w137) -> (w139:T12)
                        n328 = Build Cluster Array(w138, w136) -> (w140:T12)
                        n329 = property on="MAGNITUDE/PHASE" class="XYGraph (strict)"() -> ("Value"=w141:cluster{cluster{dbl, dbl}[]}[])  [unwired: 2 in, 2 out]
                        n330 = Bundle(w139) -> (w135:T13)  [unwired: 1 in]
                        n331 = Bundle(w140) -> (w134:T13)  [unwired: 1 in]
                        n332 = Insert Into Array(array=w141, new element #1=w135, new element #2=w134) -> (w133:cluster{cluster{dbl, dbl}[]}[])  [unwired: 1 in]
                        n333 = property on="MAGNITUDE/PHASE" class="XYGraph (strict)"("Val(Sgnl)"=w133) -> ()  [unwired: 2 in, 2 out]
                      }
                    }
                  }
                  frame #2 {
                    n334 = local read "LOOP ACT"() -> (w145:bool)
                    n335 = Select(t="VNA LOOP" ("element"), s=w145, f="WAIT" ("element")) -> (s? t:f=w144:string)
                    n336 = Enqueue Element(queue=w146, element=w144) -> ()  [unwired: 2 in, 3 out]
                    n337 = stacked-sequence {
                      frame #0 {
                        n338 = local write "ACQ Indicator"(TRUE ("ACQ Indicator")) -> ()
                      }
                      frame #1 {
                        n339 = Wait (ms)(milliseconds to wait=u32 100 ("attente (ms)")) -> ()  [unwired: 1 out]
                      }
                      frame #2 {
                        n340 = local write "ACQ Indicator"(FALSE ("ACQ Indicator")) -> ()
                      }
                    }
                  }
                }
                n341 = Wait (ms)(milliseconds to wait=u32 10 ("attente (ms)")) -> ()  [unwired: 1 out]
              }
              frame "TRACK OBS" {
                n342 = local write "STATUS"(w155) -> ()
                n343 = stacked-sequence {
                  tunnel: w152 -> [w165 _ _ _]
                  tunnel: w151 -> [w164 _ _ _]
                  tunnel: w150 -> [_ _ _ w212]
                  frame #0 {
                    n344 = local read "SPECTRUM POST PROCESSING PARAMETERS"() -> (w158:cluster{"N° SMOOTHING POINTS":i32})
                    n345 = local read "RP VNA SETTING"() -> (w178:T1)
                    n346 = Unbundle By Name(w158) -> ("N° SMOOTHING POINTS"=w157:i32)
                    n347 = Unbundle By Name(w178) -> ("Sweep size"=w177:u32)
                    n348 = local read "RAW Freq table"() -> (w173:dbl[])
                    n349 = call "VNARP-CASES.vi"("entrée d'erreur (pas d'erreur)"=w164, "Setting"=u32 0, "Énum"=T11."SWEEP START", "ID de connexion"=w165) -> ("sortie d'erreur"=w174:errorcluster, "ID de connexion en sortie"=w179:refnum<k5>)  [unwired: 3 in]
                    n350 = call "VNARP-Read.vi"("ID de connexion"=w179, "entrée d'erreur (pas d'erreur)"=w174, "SIZE"=w177) -> ("MAGNITUDE 1"=w176:sgl[], "PHASE 1"=w175:dbl[])  [unwired: 9 in, 6 out]
                    n351 = call "VNARP-BOXCAR.vi"("Y IN"=w176, "kernel size (pts)"=w157, "Freq table IN"=w173) -> ("Y OUT"=w160:dbl[], "Freq table OUT"=w172:dbl[])  [unwired: 1 in]
                    n352 = call "VNARP-BOXCAR.vi"("Y IN"=w175, "kernel size (pts)"=w157, "Freq table IN"=w173) -> ("Y OUT"=w159:dbl[], "Freq table OUT"=w161:dbl[])  [unwired: 1 in]
                    n353 = local read "VNA DATA CLUSTER"() -> (w163:T8)
                    n354 = Build Cluster Array(w172, w160) -> (w170:cluster{dbl, dbl}[])
                    n355 = Build Cluster Array(w161, w159) -> (w171:cluster{dbl, dbl}[])
                    n356 = Bundle By Name(cluster=w163, "FREQUENCY TABLE"=w161, "MAGNITUDE TABLE"=w160, "PHASE TABLE"=w159) -> (w162:T8)
                    n357 = Bundle(w170) -> (w169:cluster{cluster{dbl, dbl}[]})  [unwired: 1 in]
                    n358 = Bundle(w171) -> (w168:cluster{cluster{dbl, dbl}[]})  [unwired: 1 in]
                    n359 = Build Array(w169, w168) -> (w156:cluster{cluster{dbl, dbl}[]}[])
                    n360 = local write "MAGNITUDE/PHASE"(w156) -> ()
                    n361 = property on="MAGNITUDE/PHASE" class="XYGraph (strict)"("Val(Sgnl)"=w156) -> ()  [unwired: 2 in, 2 out]
                    n362 = local write "VNA DATA CLUSTER"(w162) -> ()
                  }
                  frame #1 {
                    n363 = local read "RP VNA SETTING"() -> (w190:T1)
                    n364 = local read "VNA DATA CLUSTER"() -> (w192:T8)
                    n365 = Unbundle By Name(w190) -> ("Sweep size"=w189:u32)
                    n366 = Max & Min(x=500 ("Fit length"), y=w189) -> (min(x,y)=w187:u32)  [unwired: 1 out]
                    n367 = Unbundle By Name(w192) -> ("FREQUENCY TABLE"=w186:ext[], "MAGNITUDE TABLE"=w185:ext[])
                    n368 = call "VNARP PARABOLA FIT.vi"("Freq Table IN"=w186, "Fit length"=w187, "Y IN"=w185) -> ("Parabol max position"=w180:dbl)  [unwired: 3 out]
                    n369 = feedback #2() -> (w191:dbl[])
                    n370 = Build Array (concatenate)(w191, w180) -> (w183:dbl[])
                    n371 = call "Search Unsorted 1D Array.vim"("element"=0.0, "unsorted 1D array"=w183) -> ("index of element"=w184:i32)  [unwired: 9 in]
                    n372 = Delete From Array(array=w183, index=w184) -> (array with subset deleted=w181:dbl[])  [unwired: 1 in, 1 out]
                    n373 = feedback-in #2(w181) -> ()
                    n374 = local write "track data"(w181) -> ()
                  }
                  frame #2 {
                    n375 = local read "TEMPORAL SMOOTHING"() -> (w195:i32)
                    n376 = local read "track data"() -> (w193:dbl[])
                    n377 = Array Size(array=w193) -> (size(s)=w197:i32)
                    n378 = Subtract(x=w197, y=w195) -> (x-y=w198:i32)
                    n379 = for {
                      N: w198 -> [_]
                      tunnel: w195 -> [w206]
                      tunnel: w193 -> [w207]
                      tunnel: [w203] -> w196 mode=indexing
                      i -> [w205]
                      n380 = Array Subset(array=w207, index=w205, length=w206) -> (w204:dbl[])
                      n381 = call-poly <vilib>:"Mean.vi"("X"=w204) -> ("mean"=w203:dbl)  [unwired: 1 out]
                    }
                    n382 = local read "N°POINTS TO DISPLAY"() -> (w199:i32)
                    n383 = Array Size(array=w196) -> (size(s)=w201:i32)
                    n384 = Subtract(x=w201, y=w199) -> (x-y=w200:i32)
                    n385 = Max & Min(x=0.0, y=w200) -> (max(x,y)=w202:dbl)  [unwired: 1 out]
                    n386 = Array Subset(array=w196, index=w202, length=w199) -> ()  [unwired: 1 out]
                  }
                  frame #3 {
                    n387 = local read "LOOP ACT"() -> (w211:bool)
                    n388 = Select(t="TRACK" ("element"), s=w211, f="WAIT" ("element")) -> (s? t:f=w210:string)
                    n389 = Enqueue Element(queue=w212, element=w210) -> ()  [unwired: 2 in, 3 out]
                  }
                }
                n390 = Wait (ms)(milliseconds to wait=u32 10 ("attente (ms)")) -> ()  [unwired: 1 out]
              }
              frame "TRACK" {
                n391 = local write "STATUS"(w217) -> ()
                n392 = stacked-sequence {
                  tunnel: w215 -> [_ w224 _]
                  tunnel: w214 -> [_ w223 _]
                  tunnel: w213 -> [_ w222 w438]
                  frame #0 {
                    n393 = local read "DELAY BETWEEN TRIG (s)"() -> (w220:i32)
                    n394 = Multiply(x=w220, y=u32 1000 ("attente (ms)")) -> (x*y=w219:u32)
                    n395 = Wait (ms)(milliseconds to wait=w219) -> ()  [unwired: 1 out]
                  }
                  frame #1 {
                    n396 = local read "CHANNELS PARAMETERS"() -> (w221:T4)
                    n397 = for {
                      tunnel: w221 -> [w230] mode=indexing
                      tunnel: w224 -> [w229]
                      tunnel: w223 -> [w228]
                      tunnel: w222 -> [w226]
                      tunnel: w221 -> [w225]
                      i -> [w227]
                      n398 = Unbundle By Name(w230) -> ("CHANNEL TRACK ?"=w231:bool)
                      n399 = case shown="True" w231 {
                        tunnel: w230 -> [_ w233]
                        tunnel: w229 -> [_ w234]
                        tunnel: w228 -> [_ w236]
                        tunnel: w227 -> [_ w235]
                        tunnel: w226 -> [_ _]
                        tunnel: w225 -> [_ w232]
                        frame False {
                        }
                        frame True {
                          n400 = stacked-sequence {
                            tunnel: w236 -> [_ w248 _ _ _ w277 w294 _ _ _ _ _ _ _]
                            tunnel: w235 -> [w237 _ _ _ w268 _ _ w316 w321 w347 _ _ _ _]
                            tunnel: w234 -> [_ w239 _ _ _ w274 w292 _ _ _ _ _ _ _]
                            tunnel: w233 -> [_ w238 _ _ w269 _ _ _ _ w341 _ _ _ _]
                            tunnel: w232 -> [_ _ _ _ w267 _ _ _ _ _ _ _ _ _]
                            frame #0 {
                              # "ATTENTION : do not trig channel choice change event !!!!"
                              # "switch"
                              n401 = local write "CHANNEL CHOICE VNA"(w237) -> ()
                              n402 = local write "CHANNELS IND TRACK"(w237) -> ()
                            }
                            frame #1 {
                              n403 = local write "VNA Settings cluster"(w238) -> ()
                              n404 = local read "RP VNA SETTING"() -> (w251:T1)
                              n405 = call "VNARP-VNASETTING CLTR MANAGMENT.vi"("VNA Settings cluster"=w238, "RP VNA SETTING"=w251) -> ("OUTPUT VNA SETTINGS"=w249:T1)  [unwired: 1 in]
                              n406 = local write "RP VNA SETTING"(w249) -> ()
                              n407 = call "VNARP-SettingsUpdate.vi"("Error IN"=w248, "RP VNA SETTINGS IN"=w249, "ID de connexion IN"=w239) -> ("Freq table"=w250:dbl[])  [unwired: 2 out]
                              n408 = local write "RAW Freq table"(w250) -> ()
                              n409 = Unbundle By Name(w238) -> ("START 2"=w241:dbl, "STOP 2"=w247:dbl, "CENTER 2"=w246:dbl, "SPAN 2"=w245:dbl, "PUMP"=w240:dbl, "PROBE"=w244:dbl, "Points N° 2"=w243:i32, "SPACING 2"=w242:dbl)
                              n410 = local write "Points N°"(w243) -> ()
                              n411 = local write "SPACING"(w242) -> ()
                              n412 = local write "CENTER"(w246) -> ()
                              n413 = local write "START"(w241) -> ()
                              n414 = local write "STOP"(w247) -> ()
                              n415 = local write "PROBE"(w244) -> ()
                              n416 = local write "SPAN"(w245) -> ()
                              n417 = local write "PUMP"(w240) -> ()
                              n418 = property on="START" class="DigNum (strict)"("Val(Sgnl)"=w241) -> ()  [unwired: 2 in, 2 out]
                              n419 = property on="PUMP" class="Slide (strict)"("Val(Sgnl)"=w240) -> ()  [unwired: 2 in, 2 out]
                            }
                            frame #2 {
                              w260 = u16 0 items=["AOUT0", "AOUT1", "AOUT2", "AOUT3"] ("Pin #")
                              w259 = u16 1 items=["AOUT0", "AOUT1", "AOUT2", "AOUT3"] ("Pin #")
                              n420 = local read "VOA Calibration cluster"() -> (w258:cluster{"PUMP":dbl[], "PROBE":dbl[]})
                              n421 = local read "NETWORK PARAMETERS"() -> (w262:T7)
                              n422 = Unbundle By Name(w262) -> ("RP-IP 2"=w261:string)
                              n423 = Unbundle By Name(w258) -> ("PUMP"=w253:dbl[], "PROBE"=w256:dbl[])
                              n424 = local read "PUMP"() -> (w254:dbl)
                              n425 = local read "PROBE"() -> (w257:dbl)
                              n426 = call "RP-VOA CONVERSION P to V.vi"("Calibration points"=w253, "% power"=w254) -> ("DAC Voltage"=w252:dbl)
                              n427 = call "RP-VOA CONVERSION P to V.vi"("Calibration points"=w256, "% power"=w257) -> ("DAC Voltage"=w255:dbl)
                              n428 = call "RP-ANALOG-OUT.vi"("Voltage"=w252, "Pin #"=w260, "IP address"=w261) -> ()  [unwired: 1 out]
                              n429 = call "RP-ANALOG-OUT.vi"("Voltage"=w255, "Pin #"=w259, "IP address"=w261) -> ()  [unwired: 1 out]
                            }
                            frame #3 {
                              n430 = local read "VNA Settings cluster"() -> (w266:T10)
                              n431 = local read "PROBE"() -> (w264:dbl)
                              n432 = local read "PUMP"() -> (w265:dbl)
                              n433 = Bundle By Name(cluster=w266, "PUMP"=w265, "PROBE"=w264) -> (w263:T10)
                              n434 = local write "VNA Settings cluster"(w263) -> ()
                            }
                            frame #4 {
                              n435 = local read "VNA Settings cluster"() -> (w272:T10)
                              n436 = Unbundle By Name(w269) -> ("CHANNEL TRACK ?"=w271:bool)
                              n437 = Bundle By Name(cluster=w272, "CHANNEL TRACK ?"=w271) -> (w270:T10)
                              n438 = Replace Array Subset(array=w267, new element=w270, index=w268) -> (w273:T4)
                              n439 = local write "CHANNELS PARAMETERS"(w273) -> ()
                            }
                            frame #5 {
                              # "wait for stab"
                              n440 = local read "DELAY AFTER SWITCH (s)"() -> (w276:i32)
                              n441 = Equal To 0?(x=w276) -> (x = 0?=w275:bool)
                              n442 = case shown="False" w275 {
                                tunnel: w277 -> [w279 _]
                                tunnel: w274 -> [w278 _]
                                frame False {
                                n443 = Tick Count (ms)() -> (millisecond timer value=w280:u32)
                                n444 = while {
                                tunnel: w280 -> [w289]
                                tunnel: w279 -> [w283]
                                tunnel: w278 -> [w282]
                                stop <- w284 stop-if-true
                                n445 = flat-sequence {
                                tunnel: w283 -> [_]
                                tunnel: w282 -> [_]
                                tunnel: [w290] -> w281
                                frame #0 {
                                }
                                frame #1 {
                                n446 = Tick Count (ms)() -> (millisecond timer value=w290:u32)
                                }
                                }
                                n447 = local read "DELAY AFTER SWITCH (s)"() -> (w288:i32)
                                n448 = Subtract(x=w281, y=w289) -> (x-y=w286:u32)
                                n449 = Multiply(x=w288, y=1000) -> (x*y=w285:i32)
                                n450 = Greater Or Equal?(x=w286, y=w285) -> (x >= y?=w284:bool)
                                }
                                }
                                frame True {
                                }
                              }
                            }
                            frame #6 {
                              # "AVERAGING IS MISSING !"
                              n451 = local read "SPECTRUM POST PROCESSING PARAMETERS"() -> (w298:cluster{"N° SMOOTHING POINTS":i32})
                              n452 = Unbundle By Name(w298) -> ("N° SMOOTHING POINTS"=w297:i32)
                              n453 = local read "RP VNA SETTING"() -> (w314:T1)
                              n454 = Unbundle By Name(w314) -> ("Sweep size"=w313:u32)
                              n455 = local read "RAW Freq table"() -> (w309:dbl[])
                              n456 = call "VNARP-CASES.vi"("entrée d'erreur (pas d'erreur)"=w294, "Setting"=u32 0, "Énum"=T11."SWEEP START", "ID de connexion"=w292) -> ("sortie d'erreur"=w310:errorcluster, "ID de connexion en sortie"=w315:refnum<k5>)  [unwired: 3 in]
                              n457 = local read "CHANNEL CHOICE VNA"() -> (w293:T3)
                              n458 = call "VNARP-Read.vi"("ID de connexion"=w315, "entrée d'erreur (pas d'erreur)"=w310, "SIZE"=w313) -> ("MAGNITUDE 1"=w312:sgl[], "PHASE 1"=w311:dbl[])  [unwired: 9 in, 6 out]
                              n459 = call "VNARP-BOXCAR.vi"("Y IN"=w312, "kernel size (pts)"=w297, "Freq table IN"=w309) -> ("Y OUT"=w300:dbl[], "Freq table OUT"=w308:dbl[])  [unwired: 1 in]
                              n460 = call "VNARP-BOXCAR.vi"("Y IN"=w311, "kernel size (pts)"=w297, "Freq table IN"=w309) -> ("Y OUT"=w299:dbl[], "Freq table OUT"=w301:dbl[])  [unwired: 1 in]
                              n461 = Build Cluster Array(w308, w300) -> (w306:cluster{dbl, dbl}[])
                              n462 = Build Cluster Array(w301, w299) -> (w307:cluster{dbl, dbl}[])
                              n463 = local read "VNA DATA CLUSTER"() -> (w303:T8)
                              n464 = Bundle By Name(cluster=w303, "CHANNEL"=w293, "FREQUENCY TABLE"=w301, "MAGNITUDE TABLE"=w300, "PHASE TABLE"=w299) -> (w302:T8)
                              n465 = Bundle(w306) -> (w305:cluster{cluster{dbl, dbl}[]})  [unwired: 1 in]
                              n466 = Bundle(w307) -> (w304:cluster{cluster{dbl, dbl}[]})  [unwired: 1 in]
                              n467 = Build Array(w305, w304) -> (w291:cluster{cluster{dbl, dbl}[]}[])
                              n468 = local write "MAGNITUDE/PHASE"(w291) -> ()
                              n469 = property on="MAGNITUDE/PHASE" class="XYGraph (strict)"("Val(Sgnl)"=w291) -> ()  [unwired: 2 in, 2 out]
                              n470 = local write "VNA DATA CLUSTER"(w302) -> ()
                            }
                            frame #7 {
                              n471 = local read "VNA DATA CLUSTER TBL"() -> (w318:T9)
                              n472 = local read "VNA DATA CLUSTER"() -> (w317:T8)
                              n473 = Replace Array Subset(array=w318, new element=w317, index=w316) -> (w319:T9)
                              n474 = local write "VNA DATA CLUSTER TBL"(w319) -> ()
                            }
                            frame #8 {
                              n475 = local read "BTN AUTOSAVE RAW DATA"() -> (w320:bool)
                              n476 = case shown="True" w320 {
                                tunnel: w321 -> [_ w323]
                                frame False {
                                }
                                frame True {
                                # "save to file vna"
                                n477 = local read "VNA DATA CLUSTER TBL"() -> (w334:T9)
                                n478 = local read "Track Repositery List"() -> (w324:path[])
                                n479 = Tick Count (ms)() -> (millisecond timer value=w332:u32)
                                n480 = Number To Decimal String(number=w332) -> (decimal integer string=w331:string)  [unwired: 1 in]
                                n481 = call "RP-VNA DATA TBL Extract.vi"("VNA DATA CLUSTER TBL"=w334, "index"=w323) -> ("appended array"=w333:ext[][])  [unwired: 2 in, 1 out]
                                n482 = Concatenate Strings("RAW VNA DATA " ("string"), w331, ".txt" ("string")) -> (w329:string)
                                n483 = Index Array(array=w324, index=w323) -> (element=w322:path)
                                n484 = Build Path(base path=w322, name or relative path=w329) -> (appended path=w328:path)
                                n485 = call-poly <vilib>:"Write Delimited Spreadsheet.vi"("file path (dialog if empty)"=w328, "format (%.3f)"="%.6f", "2D data"=w333, "transpose? (no:F)"=TRUE) -> ()  [unwired: 10 in, 2 out]
                                }
                              }
                            }
                            frame #9 {
                              # "add to track kpi tables"
                              n486 = Unbundle By Name(w341) -> ("Parafit span type"=w340:enum16{"Points N°", "Frequency", "Span %"}, "Parafit span"=w339:dbl)
                              n487 = local read "TRACK DATA CLUSTER TBL"() -> (w348:cluster{"CHANNEL":dbl, "KPI 1 TRACK":ext[]}[])
                              n488 = local read "VNA DATA CLUSTER"() -> (w356:T8)
                              n489 = local read "RP VNA SETTING"() -> (w355:T1)
                              n490 = Unbundle By Name(w355) -> ("F start"=w342:u32, "F stop"=w343:u32, "Sweep size"=w344:u32)
                              n491 = Unbundle By Name(w356) -> ("FREQUENCY TABLE"=w354:ext[], "MAGNITUDE TABLE"=w353:ext[])
                              n492 = Index Array(array=w348, index=w347) -> (element=w350:cluster{"CHANNEL":dbl, "KPI 1 TRACK":ext[]})
                              n493 = call "GET PARABOLIC FIT POINTS.vi"("Data entry"=w340, "Sweep size"=w344, "F stop"=w343, "F start"=w342, "Parabolic fit span"=w339) -> ("Points"=w345:i32)  [unwired: 6 in]
                              n494 = Unbundle By Name(w350) -> ("KPI 1 TRACK"=w352:ext[])
                              n495 = call "VNARP PARABOLA FIT.vi"("Freq Table IN"=w354, "Fit length"=w345, "Y IN"=w353) -> ("Best Polynomial Fit"=w335:dbl[], "Fit Span"=w336:dbl[], "Parabol max position"=w338:dbl, "error out"=w337:errorcluster)
                              n496 = Build Array (concatenate)(w352, w338) -> (w351:ext[])
                              n497 = case shown="No Error" w337 {
                                tunnel: w336 -> [w361 _]
                                tunnel: w335 -> [w360 _]
                                frame No Error {
                                n498 = Build Cluster Array(w361, w360) -> (w362:cluster{dbl, dbl}[])
                                n499 = property on="MAGNITUDE/PHASE" class="XYGraph (strict)"() -> ("Value"=w359:cluster{cluster{dbl, dbl}[]}[])  [unwired: 2 in, 2 out]
                                n500 = Bundle(w362) -> (w357:cluster{cluster{dbl, dbl}[]})  [unwired: 1 in]
                                n501 = Insert Into Array(array=w359, new element=w357) -> (w358:cluster{cluster{dbl, dbl}[]}[])  [unwired: 1 in]
                                n502 = property on="MAGNITUDE/PHASE" class="XYGraph (strict)"("Val(Sgnl)"=w358) -> ()  [unwired: 2 in, 2 out]
                                }
                                frame Error {
                                }
                              }
                              n503 = Bundle By Name(cluster=w350, "CHANNEL"=w347, "KPI 1 TRACK"=w351) -> (w349:cluster{"CHANNEL":dbl, "KPI 1 TRACK":ext[]})
                              n504 = Replace Array Subset(array=w348, new element=w349, index=w347) -> (w346:cluster{"CHANNEL":dbl, "KPI 1 TRACK":ext[]}[])
                              n505 = local write "TRACK DATA CLUSTER TBL"(w346) -> ()
                            }
                            frame #10 {
                              n506 = local read "TRACK DATA CLUSTER TBL"() -> (w366:cluster{"CHANNEL":dbl, "KPI 1 TRACK":ext[]}[])
                              n507 = for {
                                tunnel: w366 -> [w391] mode=indexing
                                tunnel: [w369] -> w365 mode=indexing
                                tunnel: [w368] -> w364 mode=indexing
                                tunnel: [w367] -> w363 mode=indexing
                                n508 = local read "TEMPORAL SMOOTHING"() -> (w388:i32)
                                n509 = Unbundle By Name(w391) -> ("KPI 1 TRACK"=w387:ext[])
                                n510 = Array Size(array=w387) -> (size(s)=w389:i32)
                                n511 = Subtract(x=w389, y=w388) -> (x-y=w390:i32)
                                n512 = for {
                                N: w390 -> [_]
                                tunnel: w388 -> [w395]
                                tunnel: w387 -> [w396]
                                tunnel: [w392] -> w376 mode=indexing
                                i -> [w394]
                                n513 = Array Subset(array=w396, index=w394, length=w395) -> (w393:ext[])
                                n514 = call-poly <vilib>:"Mean.vi"("X"=w393) -> ("mean"=w392:dbl)  [unwired: 1 out]
                                }
                                n515 = Delete From Array(array=w376, length=1, index=0) -> (array with subset deleted=w368:dbl[])  [unwired: 1 out]
                                n516 = local read "DISPLAY OPTION"() -> (w385:u16)
                                n517 = Index Array(array=w368, index=0) -> (element=w380:dbl)
                                n518 = local read "N°POINTS TO DISPLAY"() -> (w372:i32)
                                n519 = Subtract(x=w368, y=w380) -> (x-y=w381:dbl[])
                                n520 = Divide(x=w381, y=w380) -> (x/y=w379:dbl[])
                                n521 = Equal?(x=w385, y=u16 0) -> (x = y?=w377:bool)
                                n522 = Multiply(x=w379, y=1000000.0 ("f")) -> (x*y=w367:dbl[])
                                n523 = Select(t=w368, s=w377, f=w367) -> (s? t:f=w370:dbl[])
                                n524 = Array Size(array=w370) -> (size(s)=w374:i32)
                                n525 = Subtract(x=w374, y=w372) -> (x-y=w373:i32)
                                n526 = Max & Min(x=0.0, y=w373) -> (max(x,y)=w375:dbl)  [unwired: 1 out]
                                n527 = Array Subset(array=w370, index=w375) -> (w369:dbl[])  [unwired: 1 in]
                              }
                              n528 = local write "TRACK DATA ABS"(w364) -> ()
                              n529 = local write "TRACK DATA REL"(w363) -> ()
                              n530 = local write "LIVE TRACK"(w365) -> ()
                            }
                            frame #11 {
                              n531 = local read "TRACK DATA CLUSTER TBL"() -> (w399:cluster{"CHANNEL":dbl, "KPI 1 TRACK":ext[]}[])
                              n532 = for {
                                tunnel: w399 -> [w412] mode=indexing
                                tunnel: [w403] -> w398 mode=indexing
                                tunnel: [w402] -> w397 mode=indexing
                                n533 = Unbundle By Name(w412) -> ("KPI 1 TRACK"=w401:ext[])
                                n534 = local read "DISPLAY OPTION"() -> (w410:u16)
                                n535 = Delete From Array(array=w401, length=1, index=0) -> (array with subset deleted=w403:ext[])  [unwired: 1 out]
                                n536 = Equal?(x=w410, y=u16 0) -> ()  [unwired: 1 out]
                                n537 = Index Array(array=w403, index=0) -> (element=w405:ext)
                                n538 = Subtract(x=w403, y=w405) -> (x-y=w406:ext[])
                                n539 = Divide(x=w406, y=w405) -> (x/y=w404:ext[])
                                n540 = Multiply(x=w404, y=1000000.0 ("f")) -> (x*y=w402:ext[])
                              }
                              n541 = local write "TRACK DATA ABS NO SMOOTHING"(w398) -> ()
                              n542 = local write "TRACK DATA REL NO SMOOTHING"(w397) -> ()
                            }
                            frame #12 {
                              n543 = local read "TRACK DATA ABS NO SMOOTHING"() -> (w421:dbl[][])
                              n544 = local read "TRACK REPOSITERY"() -> (w434:path)
                              n545 = local read "TRACK REPOSITERY"() -> (w415:path)
                              n546 = local read "TRACK DATA ABS"() -> (w428:dbl[][])
                              n547 = Build Path(base path=w434, name or relative path="ALL CHANNEL ABS Track.txt") -> (appended path=w435:path)
                              n548 = Build Path(base path=w415, name or relative path="ALL CHANNEL ABS Track NS.txt") -> (appended path=w414:path)
                              n549 = call-poly <vilib>:"Write Delimited Spreadsheet.vi"("file path (dialog if empty)"=w435, "format (%.3f)"="%.6f", "2D data"=w428, "transpose? (no:F)"=TRUE) -> ()  [unwired: 10 in, 2 out]
                              n550 = call-poly <vilib>:"Write Delimited Spreadsheet.vi"("file path (dialog if empty)"=w414, "format (%.3f)"="%.6f", "2D data"=w421, "transpose? (no:F)"=TRUE) -> ()  [unwired: 10 in, 2 out]
                              n551 = local read "TRACK DATA REL NO SMOOTHING"() -> (w422:dbl[][])
                              n552 = local read "TRACK REPOSITERY"() -> (w431:path)
                              n553 = local read "TRACK REPOSITERY"() -> (w418:path)
                              n554 = local read "TRACK DATA REL"() -> (w427:dbl[][])
                              n555 = Build Path(base path=w431, name or relative path="ALL CHANNEL REL Track.txt") -> (appended path=w430:path)
                              n556 = Build Path(base path=w418, name or relative path="ALL CHANNEL REL Track NS.txt") -> (appended path=w419:path)
                              n557 = call-poly <vilib>:"Write Delimited Spreadsheet.vi"("file path (dialog if empty)"=w430, "format (%.3f)"="%.6f", "2D data"=w427, "transpose? (no:F)"=TRUE) -> ()  [unwired: 10 in, 2 out]
                              n558 = call-poly <vilib>:"Write Delimited Spreadsheet.vi"("file path (dialog if empty)"=w419, "format (%.3f)"="%.6f", "2D data"=w422, "transpose? (no:F)"=TRUE) -> ()  [unwired: 10 in, 2 out]
                            }
                            frame #13 {
                            }
                          }
                        }
                      }
                    }
                  }
                  frame #2 {
                    n559 = local read "LOOP ACT"() -> (w441:bool)
                    n560 = Select(t="TRACK" ("element"), s=w441, f="WAIT" ("element")) -> (s? t:f=w440:string)
                    n561 = Enqueue Element(queue=w438, element=w440) -> ()  [unwired: 2 in, 3 out]
                  }
                }
              }
              frame "RUN VNA" {
                n562 = local write "STATUS"(w446) -> ()
                n563 = stacked-sequence {
                  tunnel: w444 -> [w470 _ _]
                  tunnel: w443 -> [w469 _ _]
                  frame #0 {
                    n564 = local read "RP VNA SETTING"() -> (w465:T1)
                    n565 = local read "SPECTRUM POST PROCESSING PARAMETERS"() -> (w450:cluster{"N° SMOOTHING POINTS":i32})
                    n566 = Unbundle By Name(w450) -> ("N° SMOOTHING POINTS"=w448:i32)
                    n567 = Unbundle By Name(w465) -> ("Sweep size"=w464:u32)
                    n568 = local read "RAW Freq table"() -> (w460:dbl[])
                    n569 = call "VNARP-CASES.vi"("entrée d'erreur (pas d'erreur)"=w469, "Setting"=u32 0, "Énum"=T11."SWEEP START", "ID de connexion"=w470) -> ("sortie d'erreur"=w461:errorcluster, "ID de connexion en sortie"=w466:refnum<k5>)  [unwired: 3 in]
                    n570 = local read "VNA DATA CLUSTER"() -> (w454:T8)
                    n571 = call "VNARP-Read.vi"("ID de connexion"=w466, "entrée d'erreur (pas d'erreur)"=w461, "SIZE"=w464) -> ("MAGNITUDE 1"=w463:sgl[], "PHASE 1"=w462:dbl[])  [unwired: 9 in, 6 out]
                    n572 = call "VNARP-BOXCAR.vi"("Y IN"=w463, "kernel size (pts)"=w448, "Freq table IN"=w460) -> ("Y OUT"=w449:dbl[], "Freq table OUT"=w452:dbl[])  [unwired: 1 in]
                    n573 = call "VNARP-BOXCAR.vi"("Y IN"=w462, "kernel size (pts)"=w448, "Freq table IN"=w460) -> ("Y OUT"=w451:dbl[], "Freq table OUT"=w459:dbl[])  [unwired: 1 in]
                    n574 = Bundle By Name(cluster=w454, "FREQUENCY TABLE"=w452, "MAGNITUDE TABLE"=w449, "PHASE TABLE"=w451) -> (w453:T8)
                    n575 = Build Cluster Array(w452, w449) -> (w457:cluster{dbl, dbl}[])
                    n576 = Build Cluster Array(w459, w451) -> (w458:cluster{dbl, dbl}[])
                    n577 = local write "VNA DATA CLUSTER"(w453) -> ()
                    n578 = Bundle(w457) -> (w456:cluster{cluster{dbl, dbl}[]})  [unwired: 1 in]
                    n579 = Bundle(w458) -> (w455:cluster{cluster{dbl, dbl}[]})  [unwired: 1 in]
                    n580 = Build Array(w456, w455) -> (w447:cluster{cluster{dbl, dbl}[]}[])
                    n581 = local write "MAGNITUDE/PHASE"(w447) -> ()
                    n582 = property on="MAGNITUDE/PHASE" class="XYGraph (strict)"("Val(Sgnl)"=w447) -> ()  [unwired: 2 in, 2 out]
                  }
                  frame #1 {
                    n583 = local read "BTN VIEW PERSISTANCE"() -> (w471:bool)
                    n584 = case shown="True" w471 {
                      frame False {
                      }
                      frame True {
                        n585 = local read "PERSISTANCE DATA CLUSTER"() -> (w472:T8)
                        n586 = Unbundle By Name(w472) -> ("FREQUENCY TABLE"=w478:ext[], "MAGNITUDE TABLE"=w477:ext[], "PHASE TABLE"=w476:ext[])
                        n587 = property on="MAGNITUDE/PHASE" class="XYGraph (strict)"() -> ("Value"=w481:cluster{cluster{dbl, dbl}[]}[])  [unwired: 2 in, 2 out]
                        n588 = Build Cluster Array(w478, w477) -> (w479:T12)
                        n589 = Build Cluster Array(w478, w476) -> (w480:T12)
                        n590 = Bundle(w479) -> (w475:T13)  [unwired: 1 in]
                        n591 = Bundle(w480) -> (w474:T13)  [unwired: 1 in]
                        n592 = Insert Into Array(array=w481, new element #1=w475, new element #2=w474) -> (w473:cluster{cluster{dbl, dbl}[]}[])  [unwired: 1 in]
                        n593 = property on="MAGNITUDE/PHASE" class="XYGraph (strict)"("Val(Sgnl)"=w473) -> ()  [unwired: 2 in, 2 out]
                      }
                    }
                  }
                  frame #2 {
                    n594 = stacked-sequence {
                      frame #0 {
                        n595 = local write "ACQ Indicator"(TRUE ("ACQ Indicator")) -> ()
                      }
                      frame #1 {
                        n596 = Wait (ms)(milliseconds to wait=u32 100 ("attente (ms)")) -> ()  [unwired: 1 out]
                      }
                      frame #2 {
                        n597 = local write "ACQ Indicator"(FALSE ("ACQ Indicator")) -> ()
                      }
                    }
                  }
                }
                n598 = Wait (ms)(milliseconds to wait=u32 10 ("attente (ms)")) -> ()  [unwired: 1 out]
              }
              frame "CHANNEL CHANGE" {
                n599 = stacked-sequence {
                  frame #0 {
                    n600 = local read "CHANNEL CHOICE VNA"() -> (w497:T3)
                    n601 = local read "CHANNELS PARAMETERS"() -> (w498:T4)
                    n602 = Index Array(array=w498, index=w497) -> (element=w494:T10)
                    n603 = local write "VNA Settings cluster"(w494) -> ()
                    n604 = local read "RP VNA SETTING"() -> (w495:T1)
                    n605 = Unbundle By Name(w494) -> ("START 2"=w488:dbl, "STOP 2"=w493:dbl, "CENTER 2"=w492:dbl, "SPAN 2"=w491:dbl, "PUMP"=w486:dbl, "PROBE"=w487:dbl, "Points N° 2"=w490:i32, "SPACING 2"=w489:dbl)
                    n606 = local write "Points N°"(w490) -> ()
                    n607 = local write "SPACING"(w489) -> ()
                    n608 = local write "CENTER"(w492) -> ()
                    n609 = local write "START"(w488) -> ()
                    n610 = local write "STOP"(w493) -> ()
                    n611 = local write "PROBE"(w487) -> ()
                    n612 = local write "SPAN"(w491) -> ()
                    n613 = local write "PUMP"(w486) -> ()
                    n614 = call "VNARP-VNASETTING CLTR MANAGMENT.vi"("VNA Settings cluster"=w494, "RP VNA SETTING"=w495) -> ("OUTPUT VNA SETTINGS"=w496:T1)  [unwired: 1 in]
                    n615 = local write "RP VNA SETTING"(w496) -> ()
                    n616 = property on="START" class="DigNum (strict)"("Val(Sgnl)"=w488) -> ()  [unwired: 2 in, 2 out]
                  }
                  frame #1 {
                    w509 = u16 0 items=["AOUT0", "AOUT1", "AOUT2", "AOUT3"] ("Pin #")
                    w508 = u16 1 items=["AOUT0", "AOUT1", "AOUT2", "AOUT3"] ("Pin #")
                    n617 = local read "VOA Calibration cluster"() -> (w507:cluster{"PUMP":dbl[], "PROBE":dbl[]})
                    n618 = local read "NETWORK PARAMETERS"() -> (w510:T7)
                    n619 = local read "PROBE"() -> (w506:dbl)
                    n620 = Unbundle By Name(w510) -> ("RP-IP 2"=w500:string)
                    n621 = Unbundle By Name(w507) -> ("PUMP"=w501:dbl[], "PROBE"=w505:dbl[])
                    n622 = local read "PUMP"() -> (w502:dbl)
                    n623 = local read "CHANNEL CHOICE VNA"() -> (w499:T3)
                    n624 = call "RP-VOA CONVERSION P to V.vi"("Calibration points"=w501, "% power"=w502) -> ("DAC Voltage"=w503:dbl)
                    n625 = call "RP-VOA CONVERSION P to V.vi"("Calibration points"=w505, "% power"=w506) -> ("DAC Voltage"=w504:dbl)
                    n626 = call "RP-ANALOG-OUT.vi"("Voltage"=w503, "Pin #"=w509, "IP address"=w500) -> ()  [unwired: 1 out]
                    n627 = call "RP-ANALOG-OUT.vi"("Voltage"=w504, "Pin #"=w508, "IP address"=w500) -> ()  [unwired: 1 out]
                    n628 = call "RP-SWITCH CHANNEL.vi"("Channel"=w499, "IP address"=w500) -> ()  [unwired: 1 in, 1 out]
                  }
                  frame #2 {
                    n629 = local read "VNA Settings cluster"() -> (w514:T10)
                    n630 = local read "PROBE"() -> (w512:dbl)
                    n631 = local read "PUMP"() -> (w513:dbl)
                    n632 = Bundle By Name(cluster=w514, "PUMP"=w513, "PROBE"=w512) -> (w511:T10)
                    n633 = local write "VNA Settings cluster"(w511) -> ()
                  }
                  frame #3 {
                    n634 = local read "CHANNELS PARAMETERS"() -> (w520:T4)
                    n635 = local read "CHANNEL CHOICE VNA"() -> (w519:T3)
                    n636 = Index Array(array=w520, index=w519) -> (element=w518:T10)
                    n637 = local read "VNA Settings cluster"() -> (w517:T10)
                    n638 = Unbundle By Name(w518) -> ("CHANNEL TRACK ?"=w516:bool)
                    n639 = Bundle By Name(cluster=w517, "CHANNEL TRACK ?"=w516) -> (w515:T10)
                    n640 = Replace Array Subset(array=w520, new element=w515, index=w519) -> (w521:T4)
                    n641 = local write "CHANNELS PARAMETERS"(w521) -> ()
                  }
                  frame #4 {
                    n642 = local read "CHANNEL CHOICE VNA"() -> (→"CHANNEL CHOSEN":T3)
                  }
                }
              }
              frame "WAIT" {
                n643 = local write "STATUS"(w523) -> ()
              }
              frame "UPDATE" {
                n644 = local write "STATUS"(w528) -> ()
                n645 = stacked-sequence {
                  tunnel: w527 -> [w532 _ _]
                  tunnel: w526 -> [w530 _ _]
                  frame #0 {
                    n646 = local read "RP VNA SETTING"() -> (w531:T1)
                    n647 = call "VNARP-SettingsUpdate.vi"("Error IN"=w530, "RP VNA SETTINGS IN"=w531, "ID de connexion IN"=w532) -> ("Freq table"=w529:dbl[])  [unwired: 2 out]
                    n648 = local write "RAW Freq table"(w529) -> ()
                  }
                  frame #1 {
                    n649 = local read "VNA Settings cluster"() -> (w540:T10)
                    n650 = local read "Points N°"() -> (w534:i32)
                    n651 = local read "SPACING"() -> (w533:dbl)
                    n652 = local read "CENTER"() -> (w536:dbl)
                    n653 = local read "START"() -> (w539:dbl)
                    n654 = local read "SPAN"() -> (w535:dbl)
                    n655 = local read "STOP"() -> (w538:dbl)
                    n656 = Bundle By Name(cluster=w540, "START 2"=w539, "STOP 2"=w538, "CENTER 2"=w536, "SPAN 2"=w535, "Points N° 2"=w534, "SPACING 2"=w533) -> (w537:T10)
                    n657 = local write "VNA Settings cluster"(w537) -> ()
                  }
                  frame #2 {
                    n658 = local read "CHANNELS PARAMETERS"() -> (w546:T4)
                    n659 = local read "CHANNEL CHOICE VNA"() -> (w545:T3)
                    n660 = Index Array(array=w546, index=w545) -> (element=w544:T10)
                    n661 = local read "VNA Settings cluster"() -> (w543:T10)
                    n662 = Unbundle By Name(w544) -> ("CHANNEL TRACK ?"=w542:bool)
                    n663 = Bundle By Name(cluster=w543, "CHANNEL TRACK ?"=w542) -> (w541:T10)
                    n664 = Replace Array Subset(array=w546, new element=w541, index=w545) -> (w547:T4)
                    n665 = local write "CHANNELS PARAMETERS"(w547) -> ()
                  }
                }
              }
              frame "POWER UPDATE" {
                n666 = local write "STATUS"(w548) -> ()
                n667 = stacked-sequence {
                  frame #0 {
                    w558 = u16 0 items=["AOUT0", "AOUT1", "AOUT2", "AOUT3"] ("Pin #")
                    w560 = u16 1 items=["AOUT0", "AOUT1", "AOUT2", "AOUT3"] ("Pin #")
                    n668 = local read "VOA Calibration cluster"() -> (w556:cluster{"PUMP":dbl[], "PROBE":dbl[]})
                    n669 = local read "NETWORK PARAMETERS"() -> (w559:T7)
                    n670 = Unbundle By Name(w559) -> ("RP-IP 2"=w557:string)
                    n671 = Unbundle By Name(w556) -> ("PUMP"=w551:dbl[], "PROBE"=w554:dbl[])
                    n672 = local read "PUMP"() -> (w552:dbl)
                    n673 = local read "PROBE"() -> (w555:dbl)
                    n674 = call "RP-VOA CONVERSION P to V.vi"("Calibration points"=w551, "% power"=w552) -> ("DAC Voltage"=w550:dbl)
                    n675 = call "RP-VOA CONVERSION P to V.vi"("Calibration points"=w554, "% power"=w555) -> ("DAC Voltage"=w553:dbl)
                    n676 = call "RP-ANALOG-OUT.vi"("Voltage"=w553, "Pin #"=w560, "IP address"=w557) -> ()  [unwired: 1 out]
                    n677 = call "RP-ANALOG-OUT.vi"("Voltage"=w550, "Pin #"=w558, "IP address"=w557) -> ()  [unwired: 1 out]
                  }
                  frame #1 {
                    n678 = local read "VNA Settings cluster"() -> (w564:T10)
                    n679 = local read "PROBE"() -> (w562:dbl)
                    n680 = local read "PUMP"() -> (w563:dbl)
                    n681 = Bundle By Name(cluster=w564, "PUMP"=w563, "PROBE"=w562) -> (w561:T10)
                    n682 = local write "VNA Settings cluster"(w561) -> ()
                  }
                  frame #2 {
                    n683 = local read "CHANNELS PARAMETERS"() -> (w570:T4)
                    n684 = local read "CHANNEL CHOICE VNA"() -> (w569:T3)
                    n685 = Index Array(array=w570, index=w569) -> (element=w568:T10)
                    n686 = local read "VNA Settings cluster"() -> (w567:T10)
                    n687 = Unbundle By Name(w568) -> ("CHANNEL TRACK ?"=w566:bool)
                    n688 = Bundle By Name(cluster=w567, "CHANNEL TRACK ?"=w566) -> (w565:T10)
                    n689 = Replace Array Subset(array=w570, new element=w565, index=w569) -> (w571:T4)
                    n690 = local write "CHANNELS PARAMETERS"(w571) -> ()
                  }
                }
              }
              frame "SAVE VNA" {
                n691 = call "Save file"() -> ("File Name"=w572:string, "OK"=w573:bool)  [unwired: 17 in, 1 out]
                n692 = case shown="True" w573 {
                  tunnel: w572 -> [_ w575]
                  frame False {
                  }
                  frame True {
                    n693 = local read "TRACK DATA PARAMETERS"() -> (w590:cluster{"MAIN FOLDER":path})
                    n694 = Unbundle By Name(w590) -> ("MAIN FOLDER"=w589:path)
                    n695 = local read "VNA DATA CLUSTER"() -> (w585:T8)
                    n696 = Tick Count (ms)() -> (millisecond timer value=w594:u32)
                    n697 = Build Path(base path=w589, name or relative path=path "SAVED VNA SPECTRUMS ") -> (appended path=w578:path)
                    n698 = Number To Decimal String(number=w594) -> (decimal integer string=w592:string)  [unwired: 1 in]
                    n699 = call <vilib>:"Check if File or Folder Exists.vi"("path"=w578) -> ("file or folder exists?"=w577:bool, "dup path"=w576:path)  [unwired: 8 in, 1 out]
                    n700 = Unbundle By Name(w585) -> ("FREQUENCY TABLE"=w584:ext[], "MAGNITUDE TABLE"=w583:ext[], "PHASE TABLE"=w582:ext[])
                    n701 = case shown="False" w577 {
                      tunnel: [w596 w597] -> w579
                      tunnel: w576 -> [w595 w597]
                      frame False {
                        n702 = Create Folder(path (use dialog)=w595) -> (created path=w596:path)  [unwired: 2 in, 2 out]
                      }
                      frame True {
                      }
                    }
                    n703 = Concatenate Strings(w575, w592, ".txt" ("string")) -> (w591:string)
                    n704 = Build Path(base path=w579, name or relative path=w591) -> (appended path=w588:path)
                    n705 = Build Array(w584, w583, w582) -> (w581:ext[][])
                    n706 = call-poly <vilib>:"Write Delimited Spreadsheet.vi"("file path (dialog if empty)"=w588, "format (%.3f)"="%.6f", "2D data"=w581, "transpose? (no:F)"=TRUE) -> ()  [unwired: 10 in, 2 out]
                  }
                }
              }
              frame "STOP" {
                w600 = FALSE ("TRACK-STOP")
                n707 = local write "STATUS"(w599) -> ()
                n708 = local read "RP CONNECT"() -> (w598:bool)
                n709 = case shown="True" w598 {
                  tunnel: w602 -> [_ w605]
                  tunnel: w601 -> [_ w604]
                  frame False {
                  }
                  frame True {
                    n710 = TCP Close Connection(connection ID=w605, error in (no error)=w604) -> ()  [unwired: 1 in, 2 out]
                  }
                }
                n711 = local write "TRACK-STOP"(w600) -> ()
                n712 = local write "LOOP ACT"(w600) -> ()
              }
            }
          }
          frame Error {
          }
        }
      }
      n713 = And(x=w71, y=w70) -> (x .and. y?=w69:bool)
      n714 = case shown="True" w69 {
        tunnel: w80 -> [_ w84]
        tunnel: w78 -> [_ w83]
        frame False {
        }
        frame True {
          n715 = Release Queue(queue=w83, error in (no error)=w84) -> ()  [unwired: 1 in, 3 out]
          n716 = property on="MAIN TAB" class="TabCtl (strict)"("Tabs Visible?"=TRUE ("Onglets visibles ?")) -> ()  [unwired: 2 in, 2 out]
        }
      }
    }
  }
